vi "HAGAR-V.vi"() -> ()   [LabVIEW 2017]
uses:
  <vilib>/rvi/interface/nirviReadWriteControl/nirviReadWriteControl.xnode
  gvbooleschRT.vi
  <vilib>/rvi/interface/nirviCloseFPGA/nirviCloseFPGA.xnode
  GVMWHorst.vi
  GVMethodenwechsel.vi
  GVHorstSP.vi
  GVZwangs.vi
  GVHK1Hz.vi
  GVHeizenLH.vi
  GVAIs.vi
  GVTrapsMachs.vi
  GVaktuelleTDMS.vi
  GVECDs.vi
  GVZeitenZyklen.vi
  GVProbenvol.vi
  GVVentilposition.vi
  <vilib>/rvi/interface/nirviMethod/nirviMethod.xnode
  GVChroms.vi
  GVMetavariablen.vi
  GVZwangsMPV.vi
  Licor-Steuerung/HAGAR V/Licor-Steuerung/control/Emulate Licor output GV.vi
  Licor-Steuerung/HAGAR V/Licor-Steuerung/Licor-Steuerung.lvlib
  FPGA/FPGA-Programm-05-17.vi
  <vilib>/NI_Real-Time Target Support.lvlib
  <vilib>/FPGAPlugInAG/cRIO-9114/niLvFpga_WriteFifo_cRIO-9114.vi
  <vilib>/rvi/errors/niLvFpgaMergeErrorWithErrorCode.vi
  FPGA Bitfiles/HAGAR-V_FPGATarget_FPGA-Programm-05_gdVwCsZS6sg.lvbitx
  NiFpgaLv.dll
  <vilib>/Utility/error.llb/Error Cluster From Error Code.vi
  <vilib>/rvi/errors/niLvFpgaAdjustHostInterfaceError.vi
  <vilib>/FPGAPlugInAG/cRIO-9114/niLvFpga_Close_cRIO-9114.vi
  Licor-Steuerung/HAGAR V/Licor-Steuerung/control/Licor-Sequences.ctl
  Licor-Steuerung/HAGAR V/Licor-Steuerung/display/GUI_Cluster_Graph.ctl
  Licor-Steuerung/HAGAR V/Licor-Steuerung/control/Licor-Commands.ctl
  Licor-Steuerung/HAGAR V/Licor-Steuerung/control/Licor-Pump.ctl
  Licor-Steuerung/LicorLI7000/conventions/Licor-Source.ctl
  Licor-Steuerung/LicorLI7000/LicorLI7000.lvlib
  Licor-Steuerung/HAGAR V/Licor-Steuerung/control/Licor-Parameter.ctl
  Licor-Steuerung/HAGAR V/Licor-Steuerung/display/GUI_Cluster_Parameter.ctl
  Licor-Steuerung/HAGAR V/Licor-Steuerung/display/GUI_Cluster_sdv.ctl
panel:
  in  "Zyklus":enum16{"Mod0", "Mod1", "Mod2A", "Mod2B"}(ring)=enum."Mod1"
  in  "am Ende benutzen":bool
  in  "Methode speichern":bool
  out "ZyklusNummernGesamt":i32[](array[numeric])
  in  "veränderte Methode benutzen":bool
  in  "Methode verändern":bool
  out "ZyklusNummern":i32[](array[numeric])
  out "Big Ben, Methodenzeit, Zykluszeit0, Zykluszeit1, Zykluszeit2A, Zykluszeit2B":i32[](array[numeric])
  in  "global stop RT":bool
  in  "Methode":i32(ring) items=["Bedingsmethode", "Startmethode", "Meßmodus", "Shut-up-Methode", "Test", "HAG2 1/2", "Startmethode", "HAG2 1/2 Aufwärmen", "LicorDruckProfil1", "LicorDruckProfil2", "LicorDruckProfil0", "LicorDruckProfil3", "Kalibration-Meßmodus", "Kalibration-Meßmodus-II"]
  in  "Registerkarte":T1(tab)
  out "SHOK?":bool[](array[boolean])
  out "schnelle Heizungen":string[](array[string])
  out "schnelle Heizungen":dbl[](array[numeric])
  out "HorstOK?":bool[](array[boolean])
  out "AIs3OK?":bool[](array[boolean])
  out "AIs1OK?":bool[](array[boolean])
  out "AIs1":dbl[](array[numeric])
  out "AIs1":string[](array[string])
  out "AIs2":string[](array[string])
  out "AIs3":string[](array[string])
  out "AIs2":dbl[](array[numeric])
  out "AIs3":dbl[](array[numeric])
  out "Metavariablen":string[](array[string])
  out "MVWerte":dbl[](array[numeric])
  out "MWHorst":dbl[](array[numeric])
  out "HorstRegler":string[](array[string])
  out "AIs2OK?":bool[](array[boolean])
  out "Ventilposition":i32=1 min=1 max=6 step=1
  out "MVOK?":bool[](array[boolean])
  out "CPU Total (%)":dbl
  in  "MVFixwert":dbl[](array[numeric])
  in  "MVFix?":bool[](array[boolean])
  in  "LH-Gruppe":bool[](array[boolean])=[FALSE, FALSE, FALSE, FALSE, FALSE, FALSE, FALSE, FALSE, FALSE, FALSE, FALSE, FALSE]
  out "LangsameHeizungen":string[](array[string])
  out "Housekeeping1":cluster{dbl[], dbl[]}(graph)
  in  "Zeitachse1":i32(ring)=1 items=["Zykluszeit [s] Mod0", "Zykluszeit [s] Mod1", "Zykluszeit [s] Mod2A", "Zykluszeit [s] Mod2B"]
  in  "dargestellte Größe 1":i32(ring)=1 items=["T1-Spare1", "T1-Spare2", "T1-StirlingKühlkopf [°C]", "T1-PreCol1 [°C]", "T1-PreCol2 [°C]", "T1-MainCol1a [°C]", "T1-MainCol1b [°C]", "T1-MainCol2a [°C]", "T1-MainCol2b [°C]", "T1-BronkhorstUntena [°C]", "T1-BronkhorstUntenb [°C]", "T1-BronkhorstObena [°C]", "T1-BronkhorstObenb [°C]", "T1-2Pos1B [°C]", "T1-Spare9", "T1-2Pos1A [°C]", "T1-Spare10", "T1-TurboPump [°C]", "T1-StirlingPlatine [°C]", "T1-Spare5", "T1-Spare6", "T1-Spare7", "T1-Inlet [°C]", "F1-MFM-Spare", "F1-MFM0D [mL]", "P1-HeliumHP [bara]", "P1-HeliumLP [bara]", "P1-PumpVordruck [mbara]", "TurboSpeed", "I1-MS-AC [A]", "I1-Trap1 [A]", "I1-Trap2 [A]", "T2-ECD1a", "T2-ECD1b", "T2-ECD2a", "T2-ECD2b", "T2-Col1a", "T2-Col1b", "T2-Col2a", "T2-Col2b", "T2-Spare1", "T2-Spare2", "T2-Spare3", "T2-Spare4", "T2-Spare5", "T2-Spare6", "T2-Spare7", "F2-MFM2A", "F2-MFM2B", "F2-MFM2C", "P2-N2O_HP", "P2-N2O_LP", "P2-CO2_HP", "P2-CO2_LP", "AI-Spare1", "FL-MFM1000mL", "AI-Spare3", "AI-Spare4", "StirlingAlarm", "StirlingEmerg.", "AI-Spare7", "AI-Spare8", "AI-Spare9", "FL-MFM30mL", "T0-DC/DC5", "I0-24V_M0", "I0-48V_M1", "I0-24V_M1", "I0-28V_M2", "T0-Spare3", "T0-Spare2", "T0-Spare4", "T0-DC/DC7", "I0-20V_Laptop", "I0-28V_M1", "I0-24V_M2", "I0-12V_Licor", "T0-Spare1", "T0-Drier", "T0-Spare5", "F0-MFM0A [L]", "TL-Licor_a", "P0-Span-HP", "P0-spare1", "P0-Stickstoff-LP", "P0-Helium-LP", "P0-Cal-HP", "P0-P9Tavco[bar]", "F0-MFM0B [L]", "TL-Licor_b", "P0-Span-LP", "P0-spare2", "P0-Stickstoff-HP", "P0-Helium-HP", "P0-Cal-LP", "F0-MFM3", "Trap1 [°C]", "Trap2 [°C]", "PreCol1 [°C]", "PreCol2 [°C]", "MainCol1 [°C]", "MainCol2 [°C]", "PrC0 [bara]", "PrC0-Licor [bara]", "PrC1-Säule1 [bara]", "PrC1-Säule2 [bara]", "MFC1-Sample [ml/min]", "PrC1-BackFlush1 [bara]", "PrC1-BackFlush2 [bara]", "MFC1-Reaktant [l/min]", "MFC2A[ml/min]", "MFC2B[ml/min]", "MFC2C[ul/min]", "PrC2A[bara]", "MFC2D[ml/min]", "MFC2E[ml/min]", "PrC2B[bara]"]
  out "Housekeeping2":cluster{dbl[], dbl[]}(graph)
  in  "Zeitachse2":i32(ring)=1 items=["Zykluszeit [s] Mod0", "Zykluszeit [s] Mod1", "Zykluszeit [s] Mod2A", "Zykluszeit [s] Mod2B"]
  in  "dargestellte Größe 2":i32(ring)=1 items=["T1-Spare1", "T1-Spare2", "T1-StirlingKühlkopf [°C]", "T1-PreCol1 [°C]", "T1-PreCol2 [°C]", "T1-MainCol1a [°C]", "T1-MainCol1b [°C]", "T1-MainCol2a [°C]", "T1-MainCol2b [°C]", "T1-BronkhorstUntena [°C]", "T1-BronkhorstUntenb [°C]", "T1-BronkhorstObena [°C]", "T1-BronkhorstObenb [°C]", "T1-2Pos1B [°C]", "T1-Spare9", "T1-2Pos1A [°C]", "T1-Spare10", "T1-TurboPump [°C]", "T1-StirlingPlatine [°C]", "T1-Spare5", "T1-Spare6", "T1-Spare7", "T1-Inlet [°C]", "F1-MFM-Spare", "F1-MFM0D [mL]", "P1-HeliumHP [bara]", "P1-HeliumLP [bara]", "P1-PumpVordruck [mbara]", "TurboSpeed", "I1-MS-AC [A]", "I1-Trap1 [A]", "I1-Trap2 [A]", "T2-ECD1a", "T2-ECD1b", "T2-ECD2a", "T2-ECD2b", "T2-Col1a", "T2-Col1b", "T2-Col2a", "T2-Col2b", "T2-Spare1", "T2-Spare2", "T2-Spare3", "T2-Spare4", "T2-Spare5", "T2-Spare6", "T2-Spare7", "F2-MFM2A", "F2-MFM2B", "F2-MFM2C", "P2-N2O_HP", "P2-N2O_LP", "P2-CO2_HP", "P2-CO2_LP", "AI-Spare1", "FL-MFM1000mL", "AI-Spare3", "AI-Spare4", "StirlingAlarm", "StirlingEmerg.", "AI-Spare7", "AI-Spare8", "AI-Spare9", "FL-MFM30mL", "T0-DC/DC5", "I0-24V_M0", "I0-48V_M1", "I0-24V_M1", "I0-28V_M2", "T0-Spare3", "T0-Spare2", "T0-Spare4", "T0-DC/DC7", "I0-20V_Laptop", "I0-28V_M1", "I0-24V_M2", "I0-12V_Licor", "T0-Spare1", "T0-Drier", "T0-Spare5", "F0-MFM0A [L]", "TL-Licor_a", "P0-Span-HP", "P0-spare1", "P0-Stickstoff-LP", "P0-Helium-LP", "P0-Cal-HP", "P0-P9Tavco[bar]", "F0-MFM0B [L]", "TL-Licor_b", "P0-Span-LP", "P0-spare2", "P0-Stickstoff-HP", "P0-Helium-HP", "P0-Cal-LP", "F0-MFM3", "Trap1 [°C]", "Trap2 [°C]", "PreCol1 [°C]", "PreCol2 [°C]", "MainCol1 [°C]", "MainCol2 [°C]", "PrC0 [bara]", "PrC0-Licor [bara]", "PrC1-Säule1 [bara]", "PrC1-Säule2 [bara]", "MFC1-Sample [ml/min]", "PrC1-BackFlush1 [bara]", "PrC1-BackFlush2 [bara]", "MFC1-Reaktant [l/min]", "MFC2A[ml/min]", "MFC2B[ml/min]", "MFC2C[ul/min]", "PrC2A[bara]", "MFC2D[ml/min]", "MFC2E[ml/min]", "PrC2B[bara]"]
  out "Detektor 2":cluster{dbl[], dbl[]}[](graph)
  in  "Detektor":i32(ring) items=["ECD1", "ECD2"]
  in  "HK1YMin":dbl
  in  "HK1YMax":dbl=100.0
  in  "HK2YMin":dbl
  in  "HK2YMax":dbl=100.0
  in  "DetYMin":dbl
  in  "DetYMax":dbl=100.0
  in  "NeuerRefstrom":bool
  in  "RefStromECD1":i16=800 min=0 max=2500 step=1
  in  "RefStromECD2":i16=2100 min=0 max=2500 step=1
  out "schnelleAnzeige":cluster{dbl[], dbl[]}(graph)
  in  "TafelWischen!":bool
  in  "dargestellte Größe 3":i32(ring)=1 items=["Trap1 [°C]", "Trap2 [°C]", "PreCol1 [°C]", "PreCol2 [°C]", "MainCol1 [°C]", "MainCol2 [°C]", "PrC0 [bara]", "PrC0-Licor [bara]", "PrC1-Säule1 [bara]", "PrC1-Säule2 [bara]", "MFC1-Sample [ml/min]", "PrC1-BackFlush1 [bara]", "PrC1-BackFlush2 [bara]", "MFC1-Reaktant [l/min]", "MFC2A[ml/min]", "MFC2B[ml/min]", "MFC2C[ul/min]", "PrC2A[bara]", "MFC2D[ml/min]", "MFC2E[ml/min]", "PrC2B[bara]"]
  in  "An/Aus":bool
  in  "Registerkarte 2":T2(tab)
  in  "GUI_Cluster_Graph":T3={"time (global)"=0.0, "command queue"=[], "Rohdaten"=[], "Graph"={"X"=[], "Y"=[]}, "Manuelle Steuerung"={"Sequenz"=enum."test", "Manuelle Steuerung An/Aus"=FALSE}, "Sequenz out"={"sequence"=enum."WAIT", "Zeitpunkt next"=0.0, "delta t"=0.0}} caption="Cluster" {"Sequenz out"."Zeitpunkt next" format="%<%H:%M:%S%3u>T"; "time (global)" format="%<%H:%M:%S%3u\n%m/%d/%y>T"}
  in  "GUI_Cluster_Parameter":T5={"warmup (sequence)"=[{"time"=60, "Enum"=enum."wait"}], "calibrate S (sequence)"=[{"time"=60, "Enum"=enum."wait"}, {"time"=2, "Enum"=enum."getCalibrationParameter"}, {"time"=8, "Enum"=enum."calibration-S-CO2"}, {"time"=2, "Enum"=enum."getCalibrationParameter"}], "calibrate Z (sequence)"=[{"time"=60, "Enum"=enum."wait"}, {"time"=2, "Enum"=enum."getCalibrationParameter"}, {"time"=8, "Enum"=enum."calibration-Z-H2O"}, {"time"=2, "Enum"=enum."getCalibrationParameter"}, {"time"=8, "Enum"=enum."calibration-Z-CO2"}, {"time"=2, "Enum"=enum."getCalibrationParameter"}], "initialize (sequence)"=[{"time"=30, "Enum"=enum."wait"}, {"time"=2, "Enum"=enum."setPumpSlow"}, {"time"=2, "Enum"=enum."setPumpMedium"}, {"time"=2, "Enum"=enum."setPumpFast"}, {"time"=10, "Enum"=enum."initialize"}, {"time"=4, "Enum"=enum."getCalibrationParameter"}, {"time"=2, "Enum"=enum."resetH2O"}, {"time"=4, "Enum"=enum."resetCO2"}, {"time"=4, "Enum"=enum."getCalibrationParameter"}, {"time"=2, "Enum"=enum."setZeroParameter"}, {"time"=4, "Enum"=enum."getCalibrationParameter"}, {"time"=2, "Enum"=enum."setReference"}, {"time"=4, "Enum"=enum."getLicorTime"}, {"time"=5, "Enum"=enum."getInfo"}], "Licor-parameter"={"CO2 ref"=378.15, "CO2 span"=401.67, "H2O ref"=0.0, "H2O span"=0.0, "Zi"=1.2, "Zt"=6.494e-05, "Zm"=0.0, "S"=1.34, "Temp [C]"=45.0, "Pressure [hPa]"=1050.0, "Licor-Sources"=["CO2A W", "CO2B W", "H2OA W", "H2OB W", "T C", "T V", "P kPa", "P V", "RH %"], "Licor-Pump"="Off", "Zeitstempel"=timestamp(0 s since 1904-01-01)}} {"Licor-parameter"."Pressure [hPa]" format="%_5g"; "Licor-parameter"."Temp [C]" format="%.2f"; "Licor-parameter"."CO2 ref" format="%.2f"; "Licor-parameter"."CO2 span" format="%.2g"; "Licor-parameter"."H2O ref" format="%.2g"; "Licor-parameter"."H2O span" format="%.2g"; "Licor-parameter"."Zt" format="%#_4g"}
  in  "GUI_Cluster_sdv":T10={"Graph_sdv"={"X"=[], "Y"=[]}, "Breite"=20, "Berechnen"=FALSE, "residue"=0.0} {"residue" format="%_6g"}
  in  "VISA resource name":refnum<visa-resource-name>="ASRL1::INSTR" caption="VISA-Ressourcenname"
  out "TDMSwriteECD":errorcluster
  out "AIsFIFOread":errorcluster
  out "MWTrapsMachs":errorcluster
  out "TDMSwriteHK":errorcluster
  out "TDMScloseHK":errorcluster
  out "TDMSopenHK":errorcluster
  out "TDMScloseECD2":errorcluster
  out "TDMSopenECD2":errorcluster
  out "TDMScloseECD1":errorcluster
  out "TDMSopenECD1":errorcluster
  out "FIFOwriteRS485":errorcluster
  out "SerielleKomm.":errorcluster
  out "LH":errorcluster
  out "Zyklus":errorcluster
  out "ECD1dataBackup":errorcluster
  out "ECD2dataBackup":errorcluster
  # "Zyklen:   ===>>"
  # "MS"
  # "ECD1"
  # "ECD2"
  # "Zykluszeiten:   ===>>"
  # "MS"
  # "ECD1"
  # "ECD2"
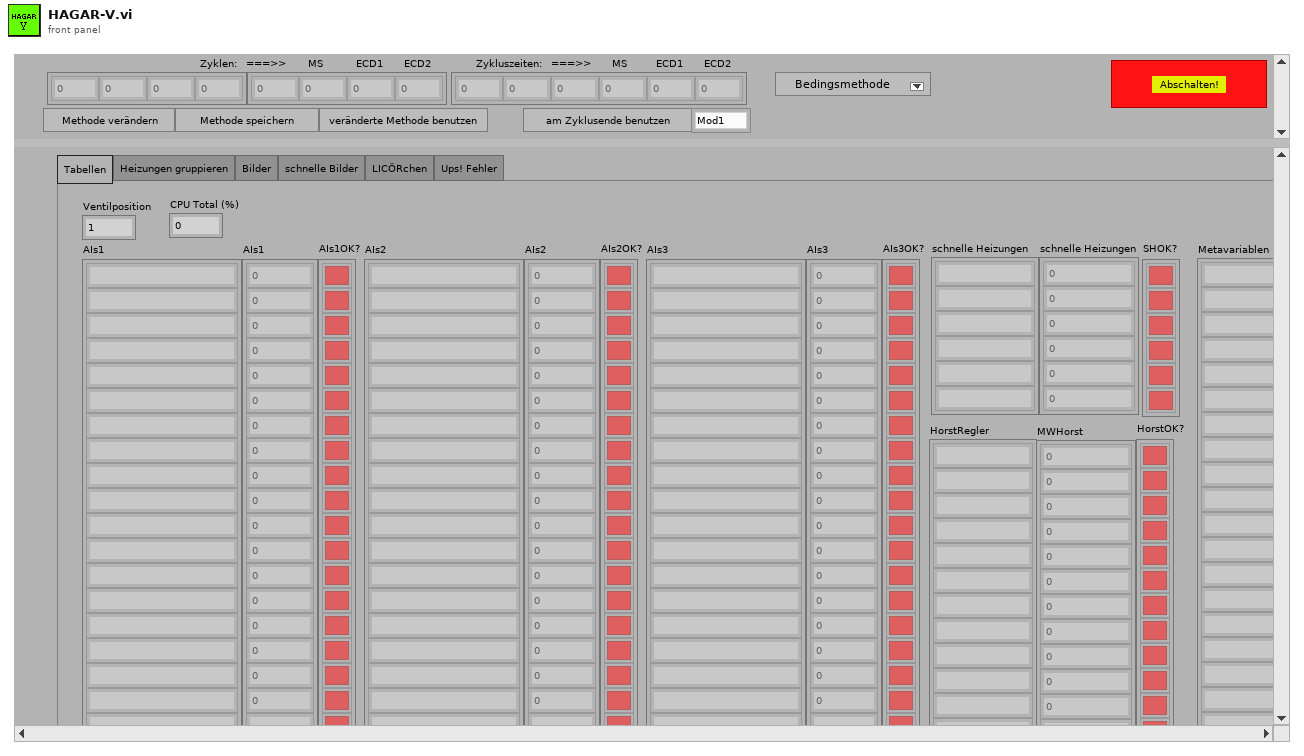
[diagram p1: front panel]
types:
  T1 = enum32{"Tabellen", "Heizungen gruppieren", "Bilder", "schnelle Bilder", "LICÖRchen", "Ups! Fehler"}
  T2 = enum32{"Graph", "Parameter / Sequenzen", "sdv", "debug"}
  T3 = typedef "Licor-Steuerung.lvlib/GUI_Cluster_Graph.ctl" = cluster{"time (global)":dbl, "command queue":cluster{"Zeit [s]":i32, "Befehl":string}[], "Rohdaten":string[], "Graph":cluster{"X":dbl[], "Y":dbl[]}, "Manuelle Steuerung":cluster{"Sequenz":T4, "Manuelle Steuerung An/Aus":bool}, "Sequenz out":cluster{"sequence":T4, "Zeitpunkt next":dbl, "delta t":dbl}}
  T4 = typedef "Licor-Steuerung.lvlib/Licor-Sequences.ctl" = enum16{"test", "WAIT", "warmup", "initialize", "calibrate Z", "calibrate S"}
  T5 = typedef "Licor-Steuerung.lvlib/GUI_Cluster_Parameter.ctl" = cluster{"warmup (sequence)":cluster{"time":i32, "Enum":T6}[], "calibrate S (sequence)":cluster{"time":i32, "Enum":T6}[], "calibrate Z (sequence)":cluster{"time":i32, "Enum":T6}[], "initialize (sequence)":cluster{"time":i32, "Enum":T6}[], "Licor-parameter":T7}
  T6 = typedef "Licor-Steuerung.lvlib/Licor-Commands.ctl" = enum16{"wait", "initialize", "resetCO2", "resetH2O", "getReference", "setReference", "calibration-Z-CO2", "calibration-Z-H2O", "calibration-S-CO2", "calibration-S-H2O", "getCalibrationParameter", "setZeroParameter", "setLicorTime", "getLicorTime", "setPumpFlowrate", "setPumpSlow", "setPumpMedium", "setPumpFast", "getInfo"}
  T7 = typedef "Licor-Steuerung.lvlib/Licor-Parameter.ctl" = cluster{"CO2 ref":dbl, "CO2 span":dbl, "H2O ref":dbl, "H2O span":dbl, "Zi":dbl, "Zt":dbl, "Zm":dbl, "S":dbl, "Temp [C]":dbl, "Pressure [hPa]":dbl, "Licor-Sources":T8[], "Licor-Pump":T9, "Zeitstempel":timestamp}
  T8 = typedef "LicorLI7000.lvlib/Licor-Source.ctl" = string
  T9 = typedef "Licor-Steuerung.lvlib/Licor-Pump.ctl" = string
  T10 = typedef "Licor-Steuerung.lvlib/GUI_Cluster_sdv.ctl" = cluster{"Graph_sdv":cluster{"X":dbl[], "Y":dbl[]}, "Breite":i32, "Berechnen":bool, "residue":dbl}
  T11 = cluster{"Zykluslängen [s]":dbl[], "ZeitpktDIOsMod0":dbl[], "ZeitpktDIOsMod1":dbl[], "ZeitpktDIOsMod2A":dbl[], "ZeitpktDIOsMod2B":dbl[], "DIOsSPMod0":bool[][], "DIOsSPMod1":bool[][], "DIOsSPMod2A":bool[][], "DIOsSPMod2B":bool[][], "Mod0HorstZeitpkt":dbl[], "Mod1HorstZeitpkt":dbl[], "Mod2AHorstZeitpkt":dbl[], "Mod2BHorstZeitpkt":dbl[], "HorstSPMod0":dbl[][], "HorstSPMod1":dbl[][], "HorstSPMod2A":dbl[][], "HorstSPMod2B":dbl[][], "LHSetpoints":dbl[], "LHHeizen?":bool[], "ZPktFPGABoolesch":dbl[], "FPGABoolesch":bool[][], "ZeitpktFPGAPID":dbl[], "FPGAPID":cluster{"d0":fxp<+/-,18,18>, "d1":fxp<+/-,21,21>}[][], "ZeitpktFPGAFixp":dbl[], dbl[][], "t_PreMach1":dbl[], "T_PreMach1":dbl[], "t_PreMach2":dbl[], "T_PreMach2":dbl[], "PIDs für \"träge\" Heizungen":cluster{"proportional gain (Kc)":dbl, "integral time (Ti, min)":dbl, "derivative time (Td, min)":dbl}[], "Zwangsbedingungen":dbl[][], "Dateien fürs MS schicken?":bool, "ZeitpunkteMPV":dbl[], "SPMPV":i32[], "ZeitpktMS-1":dbl, "ZeitpktMS-2":dbl, "Int.Start1":dbl, "Int.Stop1":dbl, "Int.Start2":dbl, "Int.Stop2":dbl, "Methodenname":string, "t_MainMach1":dbl[], "T_MainMach1":dbl[], "t_MainMach2":dbl[], "T_MainMach2":dbl[]}[]
  T12 = cluster{"DIOsMod0Nr":i32[], "DIOsMod1Nr":i32[], "DIOsMod2ANr":i32[], "DIOsMod2BNr":i32[], "AIsLH":i32[], "AnzahlRegler/Modul":i32[], "Regler für den Probenfluß":i32, "SPvorgebenMod0":string[], "SPvorgebenMod1":string[], "SPvorgebenMod2A":string[], "SPvorgebenMod2B":string[], "MWAntwortMod0":string[], "MWAntwortMod1":string[], "MWAntwortMod2A":string[], "MWAntwortMod2B":string[], "FaktorMod0":dbl[], "FaktorMod1":dbl[], "FaktorMod2A":dbl[], "FaktorMod2B":dbl[], "MWabfragenMod0":string[], "MWabfragenMod1":string[], "MWabfragenMod2A":string[], "MWabfragenMod2B":string[], "Modul1/AI koeff":dbl[][], "Modul2/AI koeff":dbl[][], "Modul3/AI koeff":dbl[][], "Traps/MachsKoeff T(R)":dbl[][], "Modul1/AIsNamen":string[], "Modul2/AIsNamen":string[], "Modul3/AIsNamen":string[], "DIOsMod0Name":string[], "DIOsMod1Name":string[], "DIOsMod2AName":string[], "DIOsMod2BName":string[], "ReglerNameMod0":string[], "ReglerNameMod1":string[], "ReglerNameMod2A":string[], "ReglerNameMod2B":string[], "Startmethode":i32, "Dateiordner Housekeeping":path, "Dateiname Housekeeping":string, "DateiordnerECD1":path, "DateinameECD1":string, "DateiordnerECD2":path, "DateinameECD2":string, "LangsameHeizungen":string[], "ModuleLH":i32[], "Metavariablen":string[], "Modul1/AI sicherer Bereich":dbl[][], "Modul2/AI sicherer Bereich":dbl[][], "Modul3/AI sicherer Bereich":dbl[][], "Traps/Machs sicherer Bereich":dbl[][], "ReglerMod0 sicherer Bereich":dbl[][], "ReglerMod1 sicherer Bereich":dbl[][], "ReglerMod2A sicherer Bereich":dbl[][], "ReglerMod2B sicherer Bereich":dbl[][], "Metavariablen grüner Bereich":dbl[][], "Traps/MachsKoeff R(U)":dbl[][], "LHGruppe":bool[]}
  T13 = enum16{"open", "replace", "create", "open or create", "replace or create", "replace or create with confirmation"}
  T14 = cluster{"Zyklus1":i32, "Zeitachse1":i32, "dargestellte Größe 1":i32, "Zyklus2":i32, "Zeitachse2":i32, "dargestellte Größe 2":i32}
  T15 = cluster{"DIOsMod0Name":string[], "DIOsMod1Name":string[], "DIOsMod2AName":string[], "DIOsMod2BName":string[], "ReglerNameMod0":string[], "ReglerNameMod1":string[], "ReglerNameMod2A":string[], "ReglerNameMod2B":string[], "LangsameHeizungen":string[]}
  T16 = cluster{"Zykluslängen [s]":dbl[], "ZeitpktDIOsMod0":dbl[], "ZeitpktDIOsMod1":dbl[], "ZeitpktDIOsMod2A":dbl[], "ZeitpktDIOsMod2B":dbl[], "DIOsSPMod0":bool[][], "DIOsSPMod1":bool[][], "DIOsSPMod2A":bool[][], "DIOsSPMod2B":bool[][], "Mod0HorstZeitpkt":dbl[], "Mod1HorstZeitpkt":dbl[], "Mod2AHorstZeitpkt":dbl[], "Mod2BHorstZeitpkt":dbl[], "HorstSPMod0":dbl[][], "HorstSPMod1":dbl[][], "HorstSPMod2A":dbl[][], "HorstSPMod2B":dbl[][], "LHSetpoints":dbl[], "LHHeizen?":bool[], "ZPktFPGABoolesch":dbl[], "FPGABoolesch":bool[][], "ZeitpktFPGAPID":dbl[], "FPGAPID":cluster{"d0":fxp<+/-,18,18>, "d1":fxp<+/-,21,21>}[][], "ZeitpktFPGAFixp":dbl[], dbl[][], "t_PreMach1":dbl[], "T_PreMach1":dbl[], "t_PreMach2":dbl[], "T_PreMach2":dbl[], "PIDs für \"träge\" Heizungen":cluster{"proportional gain (Kc)":dbl, "integral time (Ti, min)":dbl, "derivative time (Td, min)":dbl}[], "Zwangsbedingungen":dbl[][], "Dateien fürs MS schicken?":bool, "ZeitpunkteMPV":dbl[], "SPMPV":i32[], "ZeitpktMS-1":dbl, "ZeitpktMS-2":dbl, "Int.Start1":dbl, "Int.Stop1":dbl, "Int.Start2":dbl, "Int.Stop2":dbl, "Methodenname":string, "t_MainMach1":dbl[], "T_MainMach1":dbl[], "t_MainMach2":dbl[], "T_MainMach2":dbl[]}
  T17 = cluster{"Modul1/AI sicherer Bereich":dbl[][], "Modul2/AI sicherer Bereich":dbl[][], "Modul3/AI sicherer Bereich":dbl[][], "Traps/Machs sicherer Bereich":dbl[][], dbl[][], "Metavariablen grüner Bereich":dbl[][]}
  T18 = cluster{"created path":path, "created path":path}
  T19 = cluster{"created path":path, "created path":path, "created path":path, "Dateiname Housekeeping":string, "DateinameECD1":string, "DateinameECD2":string, "tdms0":refnum<k34>, "tdms1":refnum<k34>, "tdms0":refnum<k34>, "tdms1":refnum<k34>, "tdms0":refnum<k34>, "tdms1":refnum<k34>}
  T20 = cluster{"d0":fxp<+/-,18,18>, "d1":fxp<+/-,21,21>}[][]
  T21 = cluster{"proportional gain (Kc)":dbl, "integral time (Ti, min)":dbl, "derivative time (Td, min)":dbl}[]
  T22 = cluster{cluster{"ZeitpktDIOsMod2B":dbl[]}[], cluster{"DIOsSPMod2B":bool[][]}[], cluster{"Mod2BHorstZeitpkt":dbl[]}[], cluster{"HorstSPMod2B":dbl[][]}[], "LHHeizen?":bool[], "ZPktFPGABoolesch":dbl[], "FPGABoolesch":bool[][], "ZeitpktFPGAPID":dbl[], "FPGAPID":cluster{"d0":fxp<+/-,18,18>, "d1":fxp<+/-,21,21>}[][], "ZeitpktFPGAFixp":dbl[], dbl[][], "t_PreMach1":dbl[], "T_PreMach1":dbl[], "t_PreMach2":dbl[], "T_PreMach2":dbl[], "ZeitpunkteMPV":dbl[], "SPMPV":i32[], "t_MainMach1":dbl[], "T_MainMach1":dbl[], "t_MainMach2":dbl[], "T_MainMach2":dbl[]}
  T23 = cluster{"Zykluslängen [s]":dbl[], "ZeitpktDIOsMod0":dbl[], "ZeitpktDIOsMod1":dbl[], "ZeitpktDIOsMod2A":dbl[], "ZeitpktDIOsMod2B":dbl[], "DIOsSPMod0":bool[][], "DIOsSPMod1":bool[][], "DIOsSPMod2A":bool[][], "DIOsSPMod2B":bool[][], "Mod0HorstZeitpkt":dbl[], "Mod1HorstZeitpkt":dbl[], "Mod2AHorstZeitpkt":dbl[], "Mod2BHorstZeitpkt":dbl[], "HorstSPMod0":dbl[][], "HorstSPMod1":dbl[][], "HorstSPMod2A":dbl[][], "HorstSPMod2B":dbl[][], "LangsameHeizungenSP":dbl[], "LHHeizen?":bool[], "ZPktFPGABoolesch":dbl[], "FPGABoolesch":bool[][], "ZeitpktFPGAPID":dbl[], "FPGAPID":cluster{"d0":fxp<+/-,18,18>, "d1":fxp<+/-,21,21>}[][], "ZeitpktFPGAFixp":dbl[], "FPGAFixp":dbl[][], "t_PreMach1":dbl[], "T_PreMach1":dbl[], "t_PreMach2":dbl[], "T_PreMach2":dbl[], "PIDs für \"träge\" Heizungen":cluster{"proportional gain (Kc)":dbl, "integral time (Ti, min)":dbl, "derivative time (Td, min)":dbl}[], "Zwangsbedingungen":dbl[][], "MS-Daten?":bool, "ZeitpunkteMPV":dbl[], "SetpointMPV":i32[], "ZeitpktMS-1":dbl, "ZeitpktMS-2":dbl, "Int.Start1":dbl, "Int.Stop1":dbl, "Int.Start2":dbl, "Int.Stop2":dbl, "Methodenname":string, "t_MainMach1":dbl[], "T_MainMach1":dbl[], "t_MainMach2":dbl[], "T_MainMach2":dbl[]}
  T24 = cluster{"ZyklusNummern":i32[], "ZeilennummernDIOs":i32[], "ZwangsDIO?":cluster{bool[]}[], "ZeilennummernHorst":i32[], "ZwangsHorst?":cluster{bool[]}[], "ZeileFPGABoolesch":i32, "ZwangsFPGABoolesch?":bool[], "ZeileFPGAPID":i32, "ZeileFPGAFixp":i32, "ZeilePreMach1":i32, "ZeilePreMach2":i32, "ZeilennummerMPV":i32, "ZeileMainMach1":i32, "ZeileMainMach2":i32, "ZwangsMPV?":bool}
  T25 = typedef "NI_Real-Time Target Support.lvlib/RT CPU Load.ctl" = cluster{"Total (%)":dbl, "Time Critical (%)":dbl, "Timed Structures (%)":dbl, "High (%)":dbl, "Above Normal (%)":dbl, "Normal (%)":dbl, "Background (%)":dbl, "Idle (%)":dbl, "ISR (%)":dbl}
  T26 = cluster{"ZyklusNummern":i32[], i32[], "ZwangsDIO?":cluster{bool[]}[], i32[], "ZwangsHorst?":cluster{bool[]}[], i32, "ZwangsFPGABoolesch?":bool[], i32, i32, "ZeileMach":i32, "ZeileMach":i32, i32, "ZeileMach":i32, "ZeileMach":i32, "ZwangsMPV?":bool}
  T27 = cluster{string[], string[], string[], dbl[], dbl[], dbl[]}
  T28 = cluster{"Befehle1":string[], "Befehle2":string[], "Befehle3":string[]}
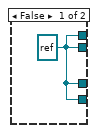
[diagram p2: hidden frame]
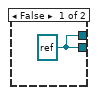
[diagram p3: hidden frame]
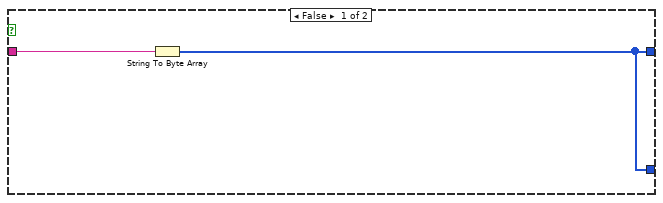
[diagram p6: hidden frame]
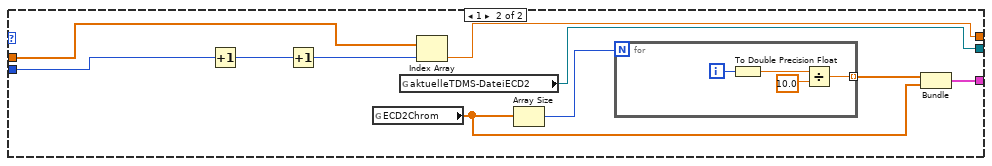
[diagram p16: hidden frame]
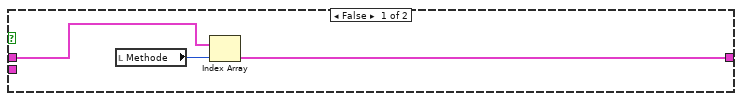
[diagram p17: hidden frame]
diagram:
  w2 = path "c:/methoden.pery" ("Datei (Dialog verwenden)")
  w3 = path "c:/einstellungen.pery" ("Datei (Dialog verwenden)")
  n1 = Open/Create/Replace File(file path (use dialog)=w3, operation (0:open)=T13."open" ("Operation (0:Öffnen)")) -> (refnum out=w15:refnum<file>)  [unwired: 4 in, 2 out]
  n2 = Open/Create/Replace File(file path (use dialog)=w2, operation (0:open)=T13."open" ("Operation (0:Öffnen)")) -> (refnum out=w11:refnum<file>)  [unwired: 4 in, 2 out]
  n3 = Read from Binary File(5:T12 {"DIOsMod0Nr"=[], "DIOsMod1Nr"=[], "DIOsMod2ANr"=[], "DIOsMod2BNr"=[], "AIsLH"=[], "AnzahlRegler/Modul"=[], "Regler für den Probenfluß"=0, "SPvorgebenMod0"=[], "SPvorgebenMod1"=[], "SPvorgebenMod2A"=[], "SPvorgebenMod2B"=[], "MWAntwortMod0"=[], "MWAntwortMod1"=[], "MWAntwortMod2A"=[], "MWAntwortMod2B"=[], "FaktorMod0"=[], "FaktorMod1"=[], "FaktorMod2A"=[], "FaktorMod2B"=[], "MWabfragenMod0"=[], "MWabfragenMod1"=[], "MWabfragenMod2A"=[], "MWabfragenMod2B"=[], "Modul1/AI koeff"=[], "Modul2/AI koeff"=[], "Modul3/AI koeff"=[], "Traps/MachsKoeff T(R)"=[], "Modul1/AIsNamen"=[], "Modul2/AIsNamen"=[], "Modul3/AIsNamen"=[], "DIOsMod0Name"=[], "DIOsMod1Name"=[], "DIOsMod2AName"=[], "DIOsMod2BName"=[], "ReglerNameMod0"=[], "ReglerNameMod1"=[], "ReglerNameMod2A"=[], "ReglerNameMod2B"=[], "Startmethode"=0, "Dateiordner Housekeeping"=path "", "Dateiname Housekeeping"="", "DateiordnerECD1"=path "", "DateinameECD1"="", "DateiordnerECD2"=path "", "DateinameECD2"="", "LangsameHeizungen"=[], "ModuleLH"=[], "Metavariablen"=[], "Modul1/AI sicherer Bereich"=[], "Modul2/AI sicherer Bereich"=[], "Modul3/AI sicherer Bereich"=[], "Traps/Machs sicherer Bereich"=[], "ReglerMod0 sicherer Bereich"=[], "ReglerMod1 sicherer Bereich"=[], "ReglerMod2A sicherer Bereich"=[], "ReglerMod2B sicherer Bereich"=[], "Metavariablen grüner Bereich"=[], "Traps/MachsKoeff R(U)"=[], "LHGruppe"=[]} ("output cluster"), 11:w15) -> (2:w13:T12, 3:w14:refnum<file>)  [unwired: 4 in, 2 out]
  n4 = Read from Binary File(5:T11 [], 11:w11) -> (2:w9:T11, 3:w10:refnum<file>)  [unwired: 4 in, 2 out]
  n5 = Close File(refnum=w14) -> ()  [unwired: 1 in, 2 out]
  n6 = Close File(refnum=w10) -> ()  [unwired: 1 in, 2 out]
  n7 = flat-sequence {
    tunnel: [w84] -> w42
    tunnel: [w145] -> w41
    tunnel: [w88] -> w39
    tunnel: [w278] -> w38
    tunnel: [w280] -> w37
    tunnel: [w272] -> w36
    tunnel: [w279] -> w35
    tunnel: [w202] -> w34
    tunnel: [w271] -> w33
    tunnel: [w270] -> w32
    tunnel: [w264] -> w31
    tunnel: [w205] -> w30
    tunnel: [w179] -> w29
    tunnel: [w277] -> w28
    tunnel: [w269] -> w27
    tunnel: [w268] -> w26
    tunnel: [w260] -> w25
    tunnel: [w259] -> w24
    tunnel: [w258] -> w23
    tunnel: [w257] -> w22
    tunnel: [w256] -> w21
    tunnel: [w255] -> w20
    tunnel: [w252] -> w19
    tunnel: [w234] -> w18
    tunnel: w13 -> [w127]
    tunnel: [w233] -> w17
    tunnel: w9 -> [w146]
    tunnel: [w145] -> w8
    tunnel: [w127] -> w7
    tunnel: [w96] -> w6
    tunnel: w3 -> [w81]
    tunnel: w2 -> [w77]
    tunnel: [w58] -> w1
    tunnel: w42 -> [w346]
    tunnel: w41 -> [w419]
    tunnel: [w346] -> w40
    tunnel: w39 -> [_]
    tunnel: w38 -> [w377]
    tunnel: w37 -> [w376]
    tunnel: w36 -> [w378]
    tunnel: w35 -> [w375]
    tunnel: w34 -> [w350]
    tunnel: w33 -> [w345]
    tunnel: w32 -> [w342]
    tunnel: w31 -> [w339]
    tunnel: w30 -> [w340]
    tunnel: w29 -> [w343]
    tunnel: w28 -> [w417]
    tunnel: w27 -> [w348]
    tunnel: w26 -> [w418]
    tunnel: w25 -> [w321]
    tunnel: w24 -> [w320]
    tunnel: w23 -> [w319]
    tunnel: w22 -> [w415]
    tunnel: w21 -> [w414]
    tunnel: w20 -> [w413]
    tunnel: w19 -> [w367]
    tunnel: w18 -> [w349]
    tunnel: w17 -> [w338]
    tunnel: w9 -> [w337]
    tunnel: w8 -> [w335]
    tunnel: w7 -> [_]
    tunnel: w6 -> [w314]
    tunnel: w1 -> [w313]
    tunnel: w40 -> [w1215]
    frame #0 {
      w54 = "config" ("string")
      w76 = string[] ["Trap1 [°C]", "Trap2 [°C]", "PreCol1 [°C]", "PreCol2 [°C]", "MainCol1 [°C]", "MainCol2 [°C]"]
      w147 = TRUE
      w161 = 0.0 ("Probenvol.1")
      w168 = dbl[] [-1.0] ("ECD1MW")
      w169 = FALSE ("ECD1Empfangen?")
      w275 = string[] ["Big Ben [s]", "Methodenzeit [s]", "Zykluszeit [s] Mod0", "Zykluszeit [s] Mod1", "Zykluszeit [s] Mod2A", "Zykluszeit [s] Mod2B"]
      w265 = FALSE ("Undefinierte Werte möglich")
      w266 = FALSE ("global stop RT")
      n8 = for {
        tunnel: [w308] -> w273 mode=indexing
        tunnel: w146 -> [w309] mode=indexing
        n9 = Unbundle(w309) -> ("Methodenname"=w308:string)  [unwired: 44 out]
      }
      n10 = Unbundle(w127) -> ("DIOsMod0Nr"=w189:i32[], "DIOsMod1Nr"=w188:i32[], "DIOsMod2ANr"=w187:i32[], "DIOsMod2BNr"=w186:i32[], "AIsLH"=w176:i32[], "AnzahlRegler/Modul"=w179:i32[], "Regler für den Probenfluß"=w233:i32, "SPvorgebenMod0"=w232:string[], "SPvorgebenMod1"=w231:string[], "SPvorgebenMod2A"=w230:string[], "SPvorgebenMod2B"=w229:string[], "MWAntwortMod0"=w228:string[], "MWAntwortMod1"=w227:string[], "MWAntwortMod2A"=w226:string[], "MWAntwortMod2B"=w225:string[], "FaktorMod0"=w224:dbl[], "FaktorMod1"=w223:dbl[], "FaktorMod2A"=w222:dbl[], "FaktorMod2B"=w221:dbl[], "MWabfragenMod0"=w220:string[], "MWabfragenMod1"=w219:string[], "MWabfragenMod2A"=w218:string[], "MWabfragenMod2B"=w217:string[], "Modul1/AI koeff"=w216:dbl[][], "Modul2/AI koeff"=w215:dbl[][], "Modul3/AI koeff"=w214:dbl[][], "Traps/MachsKoeff T(R)"=w213:dbl[][], "Modul1/AIsNamen"=w212:string[], "Modul2/AIsNamen"=w211:string[], "Modul3/AIsNamen"=w210:string[], "DIOsMod0Name"=w125:string[], "DIOsMod1Name"=w126:string[], "DIOsMod2AName"=w124:string[], "DIOsMod2BName"=w123:string[], "ReglerNameMod0"=w138:string[], "ReglerNameMod1"=w137:string[], "ReglerNameMod2A"=w136:string[], "ReglerNameMod2B"=w135:string[], "Startmethode"=w145:i32, "Dateiordner Housekeeping"=w63:path, "Dateiname Housekeeping"=w209:string, "DateiordnerECD1"=w68:path, "DateinameECD1"=w208:string, "DateiordnerECD2"=w60:path, "DateinameECD2"=w207:string, "LangsameHeizungen"=w206:string[], "ModuleLH"=w201:i32[], "Metavariablen"=w140:string[], "Modul1/AI sicherer Bereich"=w100:dbl[][], "Modul2/AI sicherer Bereich"=w99:dbl[][], "Modul3/AI sicherer Bereich"=w98:dbl[][], "Traps/Machs sicherer Bereich"=w97:dbl[][], "ReglerMod0 sicherer Bereich"=w95:dbl[][], "ReglerMod1 sicherer Bereich"=w94:dbl[][], "ReglerMod2A sicherer Bereich"=w93:dbl[][], "ReglerMod2B sicherer Bereich"=w92:dbl[][], "Metavariablen grüner Bereich"=w90:dbl[][], "LHGruppe"=w83:bool[])  [unwired: 1 out]
      "Metavariablen" <- w140
      "LangsameHeizungen" <- w206
      n11 = Initialize Array(0, 4 ("Dimension")) -> (w162:i32[])
      n12 = Initialize Array(0.0 ("Element"), 6 ("Dimension")) -> (w165:dbl[])
      n13 = global write "GVMethodenwechsel.vi" "Methodenwechsel?"(FALSE ("Methodenwechsel?")) -> ()
      n14 = local write "NeuerRefstrom"(FALSE ("NeuerRefstrom")) -> ()
      n15 = property on="dargestellte Größe 2" class="Ring (strikt)"("AllowUndefVals"=w265) -> ()  [unwired: 2 in, 2 out]
      n16 = property on="Zeitachse2" class="Ring (strikt)"("AllowUndefVals"=w265) -> ()  [unwired: 2 in, 2 out]
      n17 = property on="Zeitachse1" class="Ring (strikt)"("AllowUndefVals"=w265) -> ()  [unwired: 2 in, 2 out]
      n18 = property on="dargestellte Größe 1" class="Ring (strikt)"("AllowUndefVals"=w265) -> ()  [unwired: 2 in, 2 out]
      n19 = property on="Methode" class="Ring (strikt)"("AllowUndefVals"=w265) -> ()  [unwired: 2 in, 2 out]
      n20 = global write "GVProbenvol.vi" "Probenvol.1"(w161) -> ()
      n21 = global write "GVProbenvol.vi" "Probenvol.2"(w161) -> ()
      n22 = global write "GVECDs.vi" "ECD1MW"(w168) -> ()
      n23 = global write "GVECDs.vi" "ECD2MW"(w168) -> ()
      n24 = global write "GVECDs.vi" "ECD1Empfangen?"(w169) -> ()
      n25 = global write "GVECDs.vi" "ECD2Empfangen?"(w169) -> ()
      n26 = local write "global stop RT"(w266) -> ()
      n27 = global write "gvbooleschRT.vi" "global stop RT"(w266) -> ()
      n28 = global write "GVZeitenZyklen.vi" "ZyklusNummern"(w162) -> ()
      n29 = global write "GVZeitenZyklen.vi" "ZyklusNummernGesamt"(w162) -> ()
      n30 = global write "GVZeitenZyklen.vi" "Big Ben, Methodenzeit, Zykluszeit0, Zykluszeit1, Zykluszeit2A, Zykluszeit2B"(w165) -> ()
      n31 = property on="Methode" class="Ring (strikt)"("Value"=w145) -> ()  [unwired: 2 in, 2 out]
      n32 = Initialize Array(-1.0 ("Element"), 6 ("Dimension")) -> (w172:dbl[])
      n33 = Initialize Array(FALSE, 10 ("Dimension")) -> (w180:bool[])
      n34 = Initialize Array(-1.0 ("Element"), 96 ("Dimension")) -> (w173:dbl[])
      n35 = local write "LH-Gruppe"(w83) -> ()
      n36 = Strip Path(path=w63) -> (stripped path=w64:path)  [unwired: 1 out]
      n37 = Strip Path(path=w68) -> (stripped path=w65:path, name=w67:string)
      n38 = global write "GVZwangs.vi" "ZwangsFPGABoolesch!"(w180) -> ()
      n39 = global write "GVZwangs.vi" "ZwangsFPGABoolesch?"(w180) -> ()
      n40 = global write "GVTrapsMachs.vi" "Traps/Machs"(w172) -> ()
      n41 = global write "GVAIs.vi" "AIs"(w173) -> ()
      n42 = for {
        tunnel: w179 -> [w286] mode=indexing
        tunnel: [w283] -> w178 mode=indexing
        tunnel: [w281] -> w177 mode=indexing
        n43 = Initialize Array(0.0 ("Element"), w286) -> (w284:dbl[])
        n44 = Initialize Array(FALSE, w286) -> (w282:bool[])
        n45 = Bundle(w284) -> (w283:cluster{dbl[]})  [unwired: 1 in]
        n46 = Bundle(w282) -> (w281:cluster{bool[]})  [unwired: 1 in]
      }
      n47 = Bundle("DIOsMod0Name"=w125, "DIOsMod1Name"=w126, "DIOsMod2AName"=w124, "DIOsMod2BName"=w123, "ReglerNameMod0"=w138, "ReglerNameMod1"=w137, "ReglerNameMod2A"=w136, "ReglerNameMod2B"=w135, "LangsameHeizungen"=w206) -> (w268:T15)  [unwired: 1 in]
      n48 = Build Array (concatenate)(w138, w137, w136, w135) -> (w160:string[])
      n49 = Build Array (concatenate)(w228, w227, w226, w225) -> (w279:string[])
      n50 = Build Array (concatenate)(w232, w231, w230, w229) -> (w280:string[])
      n51 = Build Array (concatenate)(w224, w223, w222, w221) -> (w272:dbl[])
      n52 = Build Array (concatenate)(w220, w219, w218, w217) -> (w278:string[])
      n53 = Build Array (concatenate)(w138, w137, w136, w135) -> (→"HorstRegler":string[])
      n54 = Build Array (concatenate)(w95, w94, w93, w92) -> (w91:dbl[][])
      n55 = Array Size(array=w140) -> (size(s)=w75:i32)
      n56 = Build Array(w189, w188, w187, w186) -> (w185:i32[][])
      n57 = Array Size(array=w206) -> (size(s)=w205:i32)
      n58 = Add Array Elements(numeric array=w179) -> (sum=w264:i32)
      n59 = Array Size(array=w176) -> (size(s)=w175:i32)
      n60 = Index Array(array=w146, index=w145) -> (element=w144:T16)
      n61 = Add Array Elements(numeric array=w179) -> (sum=w191:i32)
      n62 = Decrement(x=w201) -> (x-1=w200:i32[])
      n63 = Build Cluster Array(w189, w188, w187, w186) -> (w271:cluster{"DIOsMod2BNr":i32[]}[])
      n64 = Build Array (concatenate)(w212, w211, w210) -> (w151:string[])
      n65 = Index Array(array=w213, index (col)=2 ("Deaktivierter Index (Spalte)")) -> (element=w260:dbl[])  [unwired: 1 in]
      n66 = Index Array(array=w213, index (col)=0 ("Deaktivierter Index (Spalte)")) -> (element=w258:dbl[])  [unwired: 1 in]
      n67 = Index Array(array=w213, index (col)=1 ("Deaktivierter Index (Spalte)")) -> (element=w259:dbl[])  [unwired: 1 in]
      n68 = Concatenate Strings("?SE0,SETP,0800" ("string"), "\n") -> (w102:string)
      n69 = Concatenate Strings("?SE0,SETP,2100" ("string"), "\n") -> (w109:string)
      n70 = Strip Path(path=w60) -> (stripped path=w59:path, name=w62:string)
      n71 = Concatenate Strings(w67, "Backup" ("string")) -> (w49:string)
      n72 = Build Path(base path=w64, name or relative path=w54) -> (appended path=w55:path)
      n73 = Build Path(base path=w65, name or relative path=w49) -> (appended path=w50:path)
      n74 = Concatenate Strings(w62, "Backup" ("string")) -> (w45:string)
      n75 = for {
        tunnel: w271 -> [w311] mode=indexing
        tunnel: [w312] -> w270 mode=indexing
        n76 = Unbundle(w311) -> ("DIOsMod2BNr"=w310:i32[])
        n77 = Array Size(array=w310) -> (size(s)=w312:i32)
      }
      n78 = property on="Methode" class="Ring (strikt)"("Strings []"=w273) -> ()  [unwired: 2 in, 2 out]
      n79 = Bundle("Modul1/AI sicherer Bereich"=w100, "Modul2/AI sicherer Bereich"=w99, "Modul3/AI sicherer Bereich"=w98, "Traps/Machs sicherer Bereich"=w97, w91, "Metavariablen grüner Bereich"=w90) -> (w96:T17)  [unwired: 1 in]
      n80 = Build Array (concatenate)(w173, w172) -> (w171:dbl[])
      n81 = Initialize Array(FALSE, w75) -> (w72:bool[])
      n82 = Array Size(array=w185) -> (size(s)=w184:i32[])
      n83 = Unbundle(w144) -> ("SPMPV"=w143:i32[])  [unwired: 44 out]
      n84 = Open/Create/Replace File(file path (use dialog)=path "c:/fromcriordy.txt" ("Dateipfad (Dialog verwenden)"), operation (0:open)=T13."replace or create" ("Operation (0:Öffnen)")) -> (refnum out=w237:refnum<file>, error out=w238:errorcluster)  [unwired: 4 in, 1 out]
      n85 = Initialize Array(0.0 ("element"), w75) -> (w73:dbl[])
      n86 = Initialize Array(0.0 ("Element"), w191) -> (w190:dbl[])
      n87 = Build Path(base path=w59, name or relative path=w45) -> (appended path=w44:path)
      n88 = Get Date/Time In Seconds() -> (seconds since 1Jan1904=w133:timestamp)
      n89 = Initialize Array(FALSE, w175) -> (w170:bool[])
      n90 = Multiply(x=w200, y=32) -> (x*y=w203:i32[])
      n91 = Initialize Array(-1.0, w191) -> (w193:dbl[])
      n92 = Array Subset(array=w151, index=32 ("Index"), length=32 ("Länge")) -> (→"AIs2":string[])
      n93 = Array Subset(array=w151, index=0 ("Index"), length=32 ("Länge")) -> (→"AIs1":string[])
      n94 = Array Subset(array=w151, index=64 ("Index"), length=32 ("Länge")) -> (→"AIs3":string[])
      n95 = global write "GVHK1Hz.vi" "Mod1Mod2Mod3/AITrapsMachs1Hz"(w171) -> ()
      n96 = global write "GVMetavariablen.vi" "Metavariablen"(w73) -> ()
      n97 = global write "GVHeizenLH.vi" "Heizen?LH"(w170) -> ()
      n98 = global write "GVZwangs.vi" "ZwangsLangsameHeizungenAn!"(w170) -> ()
      n99 = for {
        tunnel: w184 -> [w291] mode=indexing
        tunnel: [w288] -> w183 mode=indexing
        n100 = Initialize Array(FALSE, w291) -> (w289:bool[])
        n101 = Bundle(w289) -> (w288:cluster{bool[]})  [unwired: 1 in]
      }
      n102 = global write "GVHorstSP.vi" "HorstSP"(w190) -> ()
      n103 = global write "GVZwangs.vi" "ZwangsLangsameHeizungenAn?"(w170) -> ()
      n104 = global write "GVMetavariablen.vi" "MVFixwert"(w73) -> ()
      n105 = Add(x=w203, y=w176) -> (x+y=w202:i32[])
      n106 = Close File(refnum=w237, error in=w238) -> (path=w269:path)  [unwired: 1 out]
      n107 = Format Date/Time String(time format string (%c)="%Y-%m-%d--%H-%M" ("Zeitformatierungs-String (%c)"), seconds (now)=w133) -> (date/time string=w46:string)  [unwired: 1 in]
      n108 = Concatenate Strings(w49, w46) -> (w51:string)
      n109 = Concatenate Strings(w45, w46) -> (w47:string)
      n110 = Build Path(base path=w50, name or relative path=w51) -> (appended path=w48:path)
      n111 = Build Path(base path=w44, name or relative path=w47) -> (appended path=w43:path)
      n112 = Concatenate Strings(w54, w46) -> (w53:string)
      n113 = Create Folder(path (use dialog)=w48) -> (created path=w57:path)  [unwired: 2 in, 2 out]
      n114 = Create Folder(path (use dialog)=w43) -> (created path=w56:path)  [unwired: 2 in, 2 out]
      n115 = Bundle("created path"=w57, "created path"=w56) -> (w58:T18)  [unwired: 1 in]
      n116 = String To Byte Array(string=w102) -> (unsigned byte array=w104:u8[])
      n117 = String To Byte Array(string=w109) -> (unsigned byte array=w114:u8[])
      n118 = global write "GVMetavariablen.vi" "MVFix?"(w72) -> ()
      n119 = Index Array(array=w143, index=0) -> (element=w141:i32)
      n120 = Build Path(base path=w55, name or relative path=w53) -> (appended path=w52:path)
      n121 = call "FPGA-Start-15-07-17.vi"() -> ("error out"=w88:errorcluster, "FPGA VI Reference Out"=w87:refnum<k20>)  [unwired: 2 in]
      n122 = local write "MVFix?"(w72) -> ()
      n123 = local write "MVFixwert"(w73) -> ()
      n124 = global write "GVMWHorst.vi" "MWHorst"(w193) -> ()
      n125 = global write "GVVentilposition.vi" "Ventilposition"(w141) -> ()
      n126 = Build Array (concatenate)(string[] ["Jahr", "Monat", "Tag", "Stunde", "Minute", "Sekunde"] ("Array"), string[] ["Datei Nr.", "Methode Nr.", "Zyklusnr. Mod0", "Zyklusnr. Mod1", "Zyklusnr. Mod2A", "Zyklusnr. Mod2B"], w275, w151, w76, w160, "Probenvolumen1", "Probenvolumen2", "Ventilposition" ("element"), string[] ["CPU Total", "CPU Time critical", "CPU Timed Structures", "CPU High", "CPU Above normal", "CPU Normal", "CPU Background", "CPU Idle", "CPU ISR", "Memory", "SekundenTotalBrutal"]) -> (w277:string[])
      n127 = Build Array (concatenate)(w76, w160) -> (w159:string[])
      n128 = Build Array (concatenate)(w151, w76, w160) -> (w158:string[])
      n129 = Join Numbers(hi=w104, lo=u8 5) -> ((hi.lo)=w101:u16[])
      n130 = Join Numbers(hi=w114, lo=u8 6) -> ((hi.lo)=w112:u16[])
      n131 = Split 1D Array(array=w275, index=2 ("Index")) -> (second subarray=w267:string[])  [unwired: 1 out]
      n132 = Concatenate Strings("HK " ("String"), w46) -> (w120:string)
      n133 = Concatenate Strings("ECD1 " ("String"), w46) -> (w118:string)
      n134 = Concatenate Strings("ECD2 " ("String"), w46) -> (w116:string)
      n135 = property on="dargestellte Größe 1" class="Ring (strikt)"("Strings []"=w158) -> ()  [unwired: 2 in, 2 out]
      n136 = global write "GVZwangs.vi" "ZwangsHorst!"(w178) -> ()
      n137 = global write "GVZwangs.vi" "ZwangsHorst?"(w177) -> ()
      n138 = xnode "Invoke Method"("FPGA-VI-Referenz (Eingang)"=w87, "Daten"=w101) -> ("FPGA-VI-Referenz (Ausgang)"=w107:refnum<k20>)  [unwired: 2 in, 2 out]
      n139 = property on="dargestellte Größe 2" class="Ring (strikt)"("Strings []"=w158) -> ()  [unwired: 2 in, 2 out]
      n140 = property on="dargestellte Größe 3" class="Ring (strikt)"("Strings []"=w159) -> ()  [unwired: 2 in, 2 out]
      n141 = property on="Zeitachse2" class="Ring (strikt)"("Strings []"=w267) -> ()  [unwired: 2 in, 2 out]
      n142 = property on="Zeitachse1" class="Ring (strikt)"("Strings []"=w267) -> ()  [unwired: 2 in, 2 out]
      n143 = xnode "Invoke Method"("FPGA-VI-Referenz (Eingang)"=w107, "Daten"=w112) -> ("FPGA-VI-Referenz (Ausgang)"=w86:refnum<k20>)  [unwired: 2 in, 2 out]
      n144 = Create Folder(path (use dialog)=w52) -> (created path=w69:path)  [unwired: 2 in, 2 out]
      n145 = Build Path(base path=w63, name or relative path=w120) -> (appended path=w78:path)
      n146 = Build Path(base path=w68, name or relative path=w118) -> (appended path=w130:path)
      n147 = Build Path(base path=w60, name or relative path=w116) -> (appended path=w132:path)
      n148 = Strip Path(path=w81) -> (name=w80:string)  [unwired: 1 out]
      n149 = global write "GVZwangs.vi" "ZwangsDIO!"(w183) -> ()
      n150 = global write "GVZwangs.vi" "ZwangsDIO?"(w183) -> ()
      n151 = call "MPVSenden-15-07-17.vi"("Ventilposition"=0, "FPGA VI Reference In"=w86) -> ("FPGA VI Reference Out"=w84:refnum<k20>)  [unwired: 1 in, 2 out]
      n152 = Build Path(base path=w69, name or relative path=w80) -> (appended path=w71:path)
      n153 = Create Folder(path (use dialog)=w78) -> (created path=w82:path)  [unwired: 2 in, 2 out]
      n154 = Create Folder(path (use dialog)=w130) -> (created path=w129:path)  [unwired: 2 in, 2 out]
      n155 = Create Folder(path (use dialog)=w132) -> (created path=w131:path)  [unwired: 2 in, 2 out]
      n156 = Copy(10:w71, 11:w81) -> ()  [unwired: 3 in, 3 out]
      n157 = Strip Path(path=w77) -> (name=w79:string)  [unwired: 1 out]
      n158 = case shown="True" w147 {
        tunnel: [w302 w307] -> w251
        tunnel: [w302 w306] -> w250
        tunnel: w82 -> [_ w305]
        tunnel: w209 -> [_ w304]
        tunnel: w145 -> [_ w303]
        frame False {
          w302 = refnum<k34> refnum ("tdms1")
        }
        frame True {
          n159 = call "TDMS0.vi"("Startmethode"=w303, "Dateiname"=w304, "Dateiordner"=w305) -> ("tdms1"=w306:refnum<k34>, "tdms0"=w307:refnum<k34>)
          n160 = global write "GVaktuelleTDMS.vi" "aktuelleTDMS-DateiHK"(w307) -> ()
        }
      }
      n161 = case shown="True" w147 {
        tunnel: [w292 w301] -> w249
        tunnel: [w292 w300] -> w248
        tunnel: [w292 w299] -> w247
        tunnel: [w292 w298] -> w246
        tunnel: w129 -> [_ w297]
        tunnel: w208 -> [_ w296]
        tunnel: w131 -> [_ w295]
        tunnel: w207 -> [_ w294]
        tunnel: w145 -> [_ w293]
        frame False {
          w292 = refnum<k34> refnum ("tdms0")
        }
        frame True {
          n162 = call "TDMS0.vi"("Startmethode"=w293, "Dateiname"=w296, "Dateiordner"=w297) -> ("tdms1"=w300:refnum<k34>, "tdms0"=w301:refnum<k34>)
          n163 = call "TDMS0.vi"("Startmethode"=w293, "Dateiname"=w294, "Dateiordner"=w295) -> ("tdms1"=w298:refnum<k34>, "tdms0"=w299:refnum<k34>)
          n164 = global write "GVaktuelleTDMS.vi" "aktuelleTDMS-DateiECD1"(w301) -> ()
          n165 = global write "GVaktuelleTDMS.vi" "aktuelleTDMS-DateiECD2"(w299) -> ()
        }
      }
      n166 = Build Path(base path=w69, name or relative path=w79) -> (appended path=w70:path)
      n167 = Copy(10:w70, 11:w77) -> ()  [unwired: 3 in, 3 out]
      n168 = Open/Create/Replace File(file path (use dialog)=path "c:/fromcriocmd.txt" ("Pfad MS-Datei CRIO"), operation (0:open)=T13."replace or create" ("Operation (0:Öffnen)")) -> (refnum out=w243:refnum<file>, error out=w242:errorcluster)  [unwired: 4 in, 1 out]
      n169 = Write to Text File(file (use dialog)=w243, text="time=yyyymmddhhmmss\ncycle=005\ninfo=1234567890123456789012345678901234567890123456789012345678901234567890123456789012345678901234567890\nlength=100\ncmd=cycle" ("Text0 MS-Datei"), error in=w242) -> (refnum out=w240:refnum<file>, error out=w239:errorcluster)  [unwired: 1 in, 1 out]
      n170 = Bundle("created path"=w82, "created path"=w129, "created path"=w131, "Dateiname Housekeeping"=w209, "DateinameECD1"=w208, "DateinameECD2"=w207, "tdms0"=w251, "tdms1"=w250, "tdms0"=w249, "tdms1"=w248, "tdms0"=w247, "tdms1"=w246) -> (w252:T19)  [unwired: 1 in]
      n171 = call "AIKoeffSortieren.vi"("Modul3/AI koeff"=w214, "Modul2/AI koeff"=w215, "Modul1/AI koeff"=w216) -> ("P0"=w255:dbl[], "P1"=w256:dbl[], "P2"=w257:dbl[])
      n172 = Close File(refnum=w240, error in=w239) -> (path=w234:path)  [unwired: 1 out]
      "schnelle Heizungen" <- w76
    }
    frame #1 {
      w322 = dbl[] [-1.0]
      w393 = 0
      w368 = 0 ("Zyklusnummer1")
      n173 = Add Array Elements(numeric array=w342) -> (sum=w341:i32)
      n174 = Array Size(array=w350) -> (size(s)=w371:i32)
      n175 = Unbundle(w367) -> ("created path"=w366:path, "created path"=w364:path, "created path"=w363:path, "Dateiname Housekeeping"=w365:string, "DateinameECD1"=w362:string, "DateinameECD2"=w361:string, "tdms0"=w360:refnum<k34>, "tdms1"=w359:refnum<k34>, "tdms0"=w358:refnum<k34>, "tdms1"=w357:refnum<k34>, "tdms0"=w356:refnum<k34>, "tdms1"=w355:refnum<k34>)
      n176 = Index Array(array=w343, index #1=0 ("Index"), index #2=1 ("Index"), index #3=2 ("Index"), index #4=3 ("Index")) -> (element #1=w382:i32, element #2=w381:i32, element #3=w384:i32, element #4=w383:i32)
      n177 = flat-sequence {
        frame #0 {
          n178 = global write "Emulate Licor output GV.vi" "Emulator an?"(FALSE ("Emulator an?")) -> ()
        }
        frame #1 {
          n179 = control-ref of="GUI_Cluster_sdv"() -> (w421:refnum<vi>)
          n180 = control-ref of="GUI_Cluster_Graph"() -> (w423:refnum<vi>)
          n181 = control-ref of="GUI_Cluster_Parameter"() -> (w422:refnum<vi>)
          n182 = call "licore (main).vi"("GUI_Cluster_Graph (extern)"=w423, "GUI_Cluster_Parameter (extern)"=w422, "GUI_Cluster_sdv (extern)"=w421) -> ()  [unwired: 13 in]
        }
      }
      n183 = while {
        shift-right: ["Methode"] -> _
        shift-left: w419 -> [w1210]
        stop <- w1212 stop-if-true
        n184 = call "Bis zum nächsten Vielfachen warten7"("Count(mSec)"=u32 1000) -> ()  [unwired: 1 out]
        n185 = Not Equal?(x=w1210, y="Methode") -> (x != y?=w1208:bool)
        n186 = global read "gvbooleschRT.vi" "global stop RT"() -> (w1212:bool)
        n187 = global write "GVMethodenwechsel.vi" "Methodenwechsel?"(w1208) -> ()
      }
      n188 = call <vilib>:"Space Constant.vi"() -> ("String"=w328:string)
      n189 = while {
        tunnel: w346 -> [w657]
        tunnel: w415 -> [w660]
        tunnel: w414 -> [w659]
        tunnel: w413 -> [w658]
        shift-right: [w662] -> _
        shift-left: errorcluster {"status"=FALSE, "code"=0, "source"=""} ("error out") -> [w661]
        stop <- w663 stop-if-true
        n190 = call "AIsFIFORT-15-07-17.vi"("FPGA VI Reference In"=w657, "P2"=w660, "P1"=w659, "P0"=w658, "error in"=w661) -> ("error out"=w662:errorcluster)
        "AIsFIFOread" <- w662
        n191 = global read "gvbooleschRT.vi" "global stop RT"() -> (w663:bool)
      }
      n192 = while {
        tunnel: w346 -> [w664]
        tunnel: w321 -> [w667]
        tunnel: w320 -> [w666]
        tunnel: w319 -> [w665]
        shift-right: [w669] -> _
        shift-left: errorcluster {"status"=FALSE, "code"=0, "source"=""} ("error out") -> [w668]
        stop <- w671 stop-if-true
        n193 = call "Bis zum nächsten Vielfachen warten16"("Count(mSec)"=u32 100) -> ()  [unwired: 1 out]
        n194 = call "TrapsMachMitteln-15-07-17.vi"("FPGA VI Reference In"=w664, "Traps/MachKoeff2"=w667, "Traps/MachKoeff1"=w666, "Traps/MachKoeff0"=w665, "error in"=w668) -> ("error out"=w669:errorcluster)
        "MWTrapsMachs" <- w669
        n195 = global read "gvbooleschRT.vi" "global stop RT"() -> (w671:bool)
      }
      n196 = for {
        N: 1 -> [_]
        tunnel: w346 -> [w672]
        tunnel: [w672] -> w373
        n197 = call "Warten8"("Count(mSec)"=u32 100) -> ()  [unwired: 1 out]
      }
      n198 = Build Array(w328) -> (w327:string[])
      n199 = Initialize Array(-1 ("Element"), 4 ("Dimension")) -> (w344:i32[])
      n200 = global read "GVVentilposition.vi" "Ventilposition"() -> (w352:i32)
      n201 = Add(x=w384, y=w383) -> (x+y=w380:i32)
      n202 = Bundle(w327, w327, w327) -> (w391:cluster{string[], string[], string[]})  [unwired: 1 in]
      n203 = Index Array(array=w337, index=w335) -> (element=w336:T16)
      n204 = Initialize Array(cluster{"output high":dbl, "output low":dbl} {"output high"=99999.0, "output low"=0.0} ("output range"), w371) -> (w351:cluster{"output high":dbl, "output low":dbl}[])
      n205 = while {
        tunnel: w418 -> [w788]
        shift-right: [w787] -> _
        shift-left: w337 -> [w769]
        tunnel: w351 -> [w786]
        tunnel: w350 -> [w785]
        tunnel: w346 -> [w784]
        tunnel: w349 -> [w783]
        tunnel: w348 -> [w782]
        shift-right: [w776] -> _
        shift-left: 0 -> [w781]
        tunnel: w346 -> [w780]
        tunnel: w345 -> [w779]
        shift-right: [w775] -> _
        shift-left: w344 -> [w778]
        tunnel: w343 -> [w770]
        tunnel: w342 -> [w771]
        tunnel: w341 -> [w772]
        tunnel: w340 -> [w773]
        tunnel: w339 -> [w774]
        tunnel: w338 -> [w777]
        shift-right: [w693] -> _
        shift-left: w336 -> [w692]
        tunnel: w321 -> [w678]
        tunnel: w320 -> [w679]
        tunnel: w319 -> [w680]
        tunnel: w314 -> [w681]
        tunnel: w313 -> [w677]
        i -> [w696]
        stop <- w789 stop-if-true
        w686 = 0  # ZeileMainMach2
        w687 = 0  # ZeileMainMach1
        w737 = FALSE
        w736 = 0.0
        w738 = 0  # ZeilennummerMPV
        w742 = cluster{dbl[], dbl[]} {[], []}
        w751 = dbl[] []
        w755 = 0  # ZeilePreMach2
        w756 = 0  # ZeilePreMach1
        w757 = 0  # ZeileFPGAFixp
        w758 = 0  # ZeileFPGAPID
        w759 = 0  # ZeileFPGABoolesch
        w760 = i32[] [0, 0, 0, 0]  # ZeilennummernHorst
        w761 = i32[] [0, 0, 0, 0]  # ZeilennummernDIOs
        n206 = Unbundle(w677) -> ("created path"=w676:path, "created path"=w675:path)
        n207 = Unbundle(w692) -> ("Zykluslängen [s]"=w674:dbl[], "ZeitpktDIOsMod0"=w735:dbl[], "ZeitpktDIOsMod1"=w734:dbl[], "ZeitpktDIOsMod2A"=w733:dbl[], "ZeitpktDIOsMod2B"=w732:dbl[], "DIOsSPMod0"=w731:bool[][], "DIOsSPMod1"=w730:bool[][], "DIOsSPMod2A"=w729:bool[][], "DIOsSPMod2B"=w728:bool[][], "Mod0HorstZeitpkt"=w727:dbl[], "Mod1HorstZeitpkt"=w726:dbl[], "Mod2AHorstZeitpkt"=w725:dbl[], "Mod2BHorstZeitpkt"=w724:dbl[], "HorstSPMod0"=w723:dbl[][], "HorstSPMod1"=w722:dbl[][], "HorstSPMod2A"=w721:dbl[][], "HorstSPMod2B"=w720:dbl[][], "LHSetpoints"=w719:dbl[], "LHHeizen?"=w718:bool[], "ZPktFPGABoolesch"=w717:dbl[], "FPGABoolesch"=w716:bool[][], "ZeitpktFPGAPID"=w715:dbl[], "FPGAPID"=w714:T20, "ZeitpktFPGAFixp"=w713:dbl[], w712:dbl[][], "t_PreMach1"=w711:dbl[], "T_PreMach1"=w710:dbl[], "t_PreMach2"=w709:dbl[], "T_PreMach2"=w708:dbl[], "PIDs für \"träge\" Heizungen"=w707:T21, "Zwangsbedingungen"=w706:dbl[][], "Dateien fürs MS schicken?"=w705:bool, "ZeitpunkteMPV"=w704:dbl[], "SPMPV"=w703:i32[], "ZeitpktMS-1"=w702:dbl, "ZeitpktMS-2"=w701:dbl, "Int.Start1"=w700:dbl, "Int.Stop1"=w699:dbl, "Int.Start2"=w698:dbl, "Int.Stop2"=w697:dbl, "t_MainMach1"=w691:dbl[], "T_MainMach1"=w690:dbl[], "t_MainMach2"=w689:dbl[], "T_MainMach2"=w688:dbl[])  [unwired: 1 out]
        n208 = while {
          tunnel: w674 -> [w822]
          tunnel: w675 -> [w812]
          stop <- w811 stop-if-true
          n209 = global read "GVZeitenZyklen.vi" "Big Ben, Methodenzeit, Zykluszeit0, Zykluszeit1, Zykluszeit2A, Zykluszeit2B"() -> (w820:dbl[])
          n210 = Index Array(array=w820, index=5) -> (element=w818:dbl)
          n211 = global read "GVZeitenZyklen.vi" "ZyklusNummernGesamt"() -> (w823:i32[])
          n212 = call "Wait Until Next Multiple2"("Count(mSec)"=u32 100) -> ()  [unwired: 1 out]
          n213 = Index Array(array=w822, index=3) -> (element=w817:dbl)
          n214 = Subtract(x=w817, y=0.2) -> (x-y=w815:dbl)
          n215 = Greater Or Equal?(x=w818, y=w815) -> (x >= y?=w814:bool)
          n216 = global read "GVChroms.vi" "ECD2Chrom"() -> (w813:dbl[])
          n217 = case shown="True" w814 {
            tunnel: w823 -> [_ w831]
            tunnel: w813 -> [_ w830]
            tunnel: w812 -> [_ w829]
            frame False {
            }
            frame True {
              n218 = flat-sequence {
                tunnel: w831 -> [w847]
                tunnel: w830 -> [w834]
                tunnel: w829 -> [w833]
                frame #0 {
                  n219 = Index Array(array=w847, index=3) -> (element=w845:i32)
                  n220 = Number To Decimal String(number=w845, width (-)=i16 4) -> (decimal integer string=w843:string)
                  n221 = Concatenate Strings(w843, "ECD2.hag" ("string")) -> (w841:string)
                  n222 = Build Path(base path=w833, name or relative path=w841) -> (appended path=w832:path)
                  n223 = Open/Create/Replace File(file path (use dialog)=w832, operation (0:open)=T13."replace or create") -> (refnum out=w840:refnum<file>, error out=w839:errorcluster)  [unwired: 4 in, 1 out]
                  n224 = Write to Binary File(file (use dialog)=w840, data=w834, error in=w839) -> (refnum out=w838:refnum<file>, error out=w837:errorcluster)  [unwired: 3 in, 1 out]
                  n225 = Close File(refnum=w838, error in=w837) -> (error out=→"ECD2dataBackup":errorcluster)  [unwired: 1 out]
                }
                frame #1 {
                  n226 = call "Wait2"("Count(mSec)"=u32 2000) -> ()  [unwired: 1 out]
                }
              }
            }
          }
          n227 = global read "GVMethodenwechsel.vi" "Methodenwechsel?"() -> (w826:bool)
          n228 = global read "gvbooleschRT.vi" "global stop RT"() -> (w827:bool)
          n229 = Or(x=w826, y=w827) -> (x .or. y?=w828:bool)
          n230 = local read "veränderte Methode benutzen"() -> (w825:bool)
          n231 = Or(x=w828, y=w825) -> (x .or. y?=w811:bool)
        }
        n232 = while {
          tunnel: w674 -> [w859]
          tunnel: w676 -> [w849]
          stop <- w863 stop-if-true
          n233 = global read "GVZeitenZyklen.vi" "Big Ben, Methodenzeit, Zykluszeit0, Zykluszeit1, Zykluszeit2A, Zykluszeit2B"() -> (w857:dbl[])
          n234 = Index Array(array=w857, index=4) -> (element=w855:dbl)
          n235 = global read "GVZeitenZyklen.vi" "ZyklusNummernGesamt"() -> (w860:i32[])
          n236 = call "Wait Until Next Multiple"("Count(mSec)"=u32 100) -> ()  [unwired: 1 out]
          n237 = Index Array(array=w859, index=2) -> (element=w854:dbl)
          n238 = Subtract(x=w854, y=0.2) -> (x-y=w852:dbl)
          n239 = Greater Or Equal?(x=w855, y=w852) -> (x >= y?=w851:bool)
          n240 = global read "GVChroms.vi" "ECD1Chrom"() -> (w850:dbl[])
          n241 = case shown="True" w851 {
            tunnel: w860 -> [_ w869]
            tunnel: w850 -> [_ w868]
            tunnel: w849 -> [_ w867]
            frame False {
            }
            frame True {
              n242 = flat-sequence {
                tunnel: w869 -> [w885]
                tunnel: w868 -> [w872]
                tunnel: w867 -> [w871]
                frame #0 {
                  n243 = Index Array(array=w885, index=2) -> (element=w883:i32)
                  n244 = Number To Decimal String(number=w883, width (-)=i16 4) -> (decimal integer string=w881:string)
                  n245 = Concatenate Strings(w881, "ECD1.hag" ("string")) -> (w879:string)
                  n246 = Build Path(base path=w871, name or relative path=w879) -> (appended path=w870:path)
                  n247 = Open/Create/Replace File(file path (use dialog)=w870, operation (0:open)=T13."replace or create") -> (refnum out=w878:refnum<file>, error out=w877:errorcluster)  [unwired: 4 in, 1 out]
                  n248 = Write to Binary File(file (use dialog)=w878, data=w872, error in=w877) -> (refnum out=w876:refnum<file>, error out=w875:errorcluster)  [unwired: 3 in, 1 out]
                  n249 = Close File(refnum=w876, error in=w875) -> (error out=→"ECD1dataBackup":errorcluster)  [unwired: 1 out]
                }
                frame #1 {
                  n250 = call "Wait"("Count(mSec)"=u32 2000) -> ()  [unwired: 1 out]
                }
              }
            }
          }
          n251 = global read "GVMethodenwechsel.vi" "Methodenwechsel?"() -> (w864:bool)
          n252 = global read "gvbooleschRT.vi" "global stop RT"() -> (w865:bool)
          n253 = Or(x=w864, y=w865) -> (x .or. y?=w866:bool)
          n254 = local read "veränderte Methode benutzen"() -> (w862:bool)
          n255 = Or(x=w866, y=w862) -> (x .or. y?=w863:bool)
        }
        n256 = Add(x=w778, y=1) -> (x+y=w746:i32[])
        n257 = local read "Methode"() -> (w695:i32)
        n258 = Build Cluster Array(w731, w730, w729, w728) -> (w765:cluster{"DIOsSPMod2B":bool[][]}[])
        n259 = Build Cluster Array(w723, w722, w721, w720) -> (w763:cluster{"HorstSPMod2B":dbl[][]}[])
        n260 = Build Cluster Array(w735, w734, w733, w732) -> (w766:cluster{"ZeitpktDIOsMod2B":dbl[]}[])
        n261 = Build Cluster Array(w727, w726, w725, w724) -> (w764:cluster{"Mod2BHorstZeitpkt":dbl[]}[])
        n262 = Equal?(x=w696, y=0) -> (x = y?=w767:bool)
        n263 = while {
          tunnel: w674 -> [w797]
          stop <- w800 stop-if-true
          n264 = global read "GVZeitenZyklen.vi" "Big Ben, Methodenzeit, Zykluszeit0, Zykluszeit1, Zykluszeit2A, Zykluszeit2B"() -> (w806:dbl[])
          n265 = To Long Integer(number="Zyklus") -> (32bit integer=w792:i32)
          n266 = Index Array(array=w797, index=w792) -> (element=w796:dbl)
          n267 = Subtract(x=w796, y=1.0) -> (x-y=w794:dbl)
          n268 = Add(x=w792, y=2) -> (x+y=w790:i32)
          n269 = call "Wait3"("Count(mSec)"=u32 100) -> ()  [unwired: 1 out]
          n270 = global read "GVMethodenwechsel.vi" "Methodenwechsel?"() -> (w802:bool)
          n271 = global read "gvbooleschRT.vi" "global stop RT"() -> (w803:bool)
          n272 = local read "am Ende benutzen"() -> (w805:bool)
          n273 = local read "veränderte Methode benutzen"() -> (w798:bool)
          n274 = Index Array(array=w806, index=w790) -> (element=w807:dbl)
          n275 = Or(x=w802, y=w803) -> (x .or. y?=w801:bool)
          n276 = Greater Or Equal?(x=w807, y=w794) -> (x >= y?=w808:bool)
          n277 = And(x=w808, y=w805) -> (x .and. y?=w799:bool)
          n278 = case shown="True" w799 {
            frame False {
            }
            frame True {
              n279 = local write "veränderte Methode benutzen"(TRUE ("veränderte Methode benutzen")) -> ()
              n280 = local write "am Ende benutzen"(FALSE ("am Ende benutzen")) -> ()
            }
          }
          n281 = Or(x=w801, y=w798) -> (x .or. y?=w800:bool)
        }
        n282 = while {
          tunnel: w771 -> [w955]
          tunnel: w774 -> [w948]
          tunnel: w773 -> [w949]
          tunnel: w770 -> [w954]
          tunnel: w772 -> [w950]
          tunnel: w706 -> [w951]
          stop <- w957 stop-if-true
          n283 = call "Bis zum nächsten Vielfachen warten10"("Count(mSec)"=u32 1000) -> ()  [unwired: 1 out]
          n284 = local read "Methode"() -> (w953:i32)
          n285 = global read "GVMethodenwechsel.vi" "Methodenwechsel?"() -> (w959:bool)
          n286 = global read "gvbooleschRT.vi" "global stop RT"() -> (w960:bool)
          n287 = case shown="True" "global stop RT" {
            frame False {
            }
            frame True {
              n288 = global write "gvbooleschRT.vi" "global stop RT"(TRUE ("global stop RT")) -> ()
            }
          }
          n289 = call "ZwangsbedingungenGV-15-07-17.vi"("AnzahlHorst"=w948, "AnzahlHorst/Modul"=w954, "AnzahlLH"=w949, "AnzahlDIOs/Modul"=w955, "AnzahlDIOs"=w950, "Zwangsbedingungen"=w951, "Methodennummer"=w953) -> ("Methodennummer"=w952:i32)  [unwired: 4 in]
          n290 = local write "Methode"(w952) -> ()
          n291 = local read "veränderte Methode benutzen"() -> (w958:bool)
          n292 = Compound Arithmetic op=OR(w960, w959, w958) -> (w957:bool)
        }
        n293 = global read "GVZeitenZyklen.vi" "ZyklusNummern"() -> (w745:i32[])
        n294 = global read "GVZwangs.vi" "ZwangsHorst?"() -> (w750:cluster{bool[]}[])
        n295 = global read "gvbooleschRT.vi" "global stop RT"() -> (w789:bool)
        n296 = global read "GVZwangsMPV.vi" "ZwangsMPV?"() -> (w684:bool)
        n297 = global read "GVZwangs.vi" "ZwangsDIO?"() -> (w749:cluster{bool[]}[])
        n298 = global read "GVaktuelleTDMS.vi" "aktuelleTDMS-DateiECD1"() -> (w744:refnum<k34>)
        n299 = Bundle(w766, w765, w764, w763, "LHHeizen?"=w718, "ZPktFPGABoolesch"=w717, "FPGABoolesch"=w716, "ZeitpktFPGAPID"=w715, "FPGAPID"=w714, "ZeitpktFPGAFixp"=w713, w712, "t_PreMach1"=w711, "T_PreMach1"=w710, "t_PreMach2"=w709, "T_PreMach2"=w708, "ZeitpunkteMPV"=w704, "SPMPV"=w703, "t_MainMach1"=w691, "T_MainMach1"=w690, "t_MainMach2"=w689, "T_MainMach2"=w688) -> (w762:T22)  [unwired: 1 in]
        n300 = Index Array(array=w769, index=w695) -> (element=w694:T16)
        n301 = global read "GVZwangs.vi" "ZwangsFPGABoolesch?"() -> (w748:bool[])
        n302 = while {
          tunnel: w785 -> [w938]
          tunnel: w786 -> [w941]
          tunnel: w784 -> [w942]
          tunnel: w719 -> [w939]
          tunnel: w707 -> [w940]
          shift-right: [w936] -> _
          shift-left: errorcluster {"status"=FALSE, "code"=0, "source"=""} ("error out") -> [w937]
          stop <- w943 stop-if-true
          n303 = call "LH-15-07-17.vi"("FPGA VI Reference In"=w942, "OutputRange"=w941, "LHSetpoints"=w939, "AIsLH"=w938, "error in"=w937, "LH-Gruppe"="LH-Gruppe", "PIDs für \"träge\" Heizungen"=w940) -> ("error out"=w936:errorcluster)
          "LH" <- w936
          n304 = call "Bis zum nächsten Vielfachen warten12"("Count(mSec)"=u32 100) -> ()  [unwired: 1 out]
          n305 = global read "GVMethodenwechsel.vi" "Methodenwechsel?"() -> (w945:bool)
          n306 = global read "gvbooleschRT.vi" "global stop RT"() -> (w946:bool)
          n307 = local read "veränderte Methode benutzen"() -> (w944:bool)
          n308 = Compound Arithmetic op=OR(w946, w945, w944) -> (w943:bool)
        }
        n309 = while {
          shift-right: [w899] -> _
          shift-left: w737 -> [w903]
          shift-right: [w898] -> _
          shift-left: w736 -> [w902]
          shift-right: [w897] -> _
          shift-left: w737 -> [w901]
          shift-right: [w896] -> _
          shift-left: w736 -> [w900]
          tunnel: w777 -> [w895]
          tunnel: w700 -> [w890]
          tunnel: w699 -> [w889]
          tunnel: w698 -> [w888]
          tunnel: w697 -> [w887]
          stop <- w892 stop-if-true
          n310 = call "Integrieren.vi"("Integrieren1"=w903, "Integral1"=w902, "Integrieren2"=w901, "Integral2"=w900, "Int.Start1"=w890, "Int.Stop1"=w889, "Int.Start2"=w888, "HorstProbenflußNr."=w895, "Int.Stop2"=w887) -> ("Integrieren1"=w899:bool, "Integral1"=w898:dbl, "Integrieren2"=w897:bool, "Integral2"=w896:dbl)  [unwired: 7 in]
          n311 = call "Bis zum nächsten Vielfachen warten9"("Count(mSec)"=u32 100) -> ()  [unwired: 1 out]
          n312 = global read "GVMethodenwechsel.vi" "Methodenwechsel?"() -> (w893:bool)
          n313 = global read "gvbooleschRT.vi" "global stop RT"() -> (w894:bool)
          n314 = local read "veränderte Methode benutzen"() -> (w891:bool)
          n315 = Compound Arithmetic op=OR(w894, w893, w891) -> (w892:bool)
        }
        n316 = while "Zeit" {
          tunnel: w767 -> [w1147]
          tunnel: w674 -> [w1145]
          tunnel: w746 -> [w1140]
          tunnel: [w1139] -> w775
          shift-right: [w1136] -> _
          shift-left: 0.0 -> [w1137]
          i -> [w1149]
          stop <- w1142 stop-if-true
          n317 = Equal?(x=w1149, y=0) -> (x = y?=w1138:bool)
          n318 = call "Bis zum nächsten Vielfachen warten15"("Count(mSec)"=u32 50) -> ()  [unwired: 1 out]
          n319 = call "BigBen-01-16.vi"("MethodenStartzeit"=w1137, "Methodenstart?"=w1138, "Programmstart?"=w1147, "Zykluslängen [s]"=w1145, "MethodenStartZyklusNummern"=w1140) -> ("MethodenStartzeit"=w1136:dbl, "ZyklusNummernGesamt"=w1139:i32[])  [unwired: 2 in]
          n320 = global read "GVMethodenwechsel.vi" "Methodenwechsel?"() -> (w1141:bool)
          n321 = global read "gvbooleschRT.vi" "global stop RT"() -> (w1146:bool)
          n322 = Or(x=w1141, y=w1146) -> (x .or. y?=w1143:bool)
          n323 = local read "veränderte Methode benutzen"() -> (w1144:bool)
          n324 = Or(x=w1144, y=w1143) -> (x .or. y?=w1142:bool)
        }
        n325 = Bundle(w751, w751, w751, w751) -> (w752:cluster{dbl[], dbl[], dbl[], dbl[]})  [unwired: 1 in]
        n326 = while {
          tunnel: w788 -> [w1162]
          shift-right: [w1153] -> _
          shift-left: w694 -> [w1161]
          tunnel: w695 -> [w1159]
          shift-right: [w1151] -> w787
          shift-left: w769 -> [w1160]
          tunnel: [w1152] -> w693
          stop <- w1155 stop-if-true
          n327 = call "Bis zum nächsten Vielfachen warten8"("Count(mSec)"=u32 500) -> ()  [unwired: 1 out]
          n328 = global read "GVMethodenwechsel.vi" "Methodenwechsel?"() -> (w1157:bool)
          n329 = global read "gvbooleschRT.vi" "global stop RT"() -> (w1156:bool)
          n330 = case shown="True" "Methode verändern" {
            tunnel: w1162 -> [_ w1184]
            tunnel: w1161 -> [w1181 w1183]
            tunnel: [w1181 w1182] -> w1153
            frame False {
            }
            frame True {
              n331 = call "methodeändern-15-07-17.vi"("->Methode"=w1183, "Namen"=w1184) -> ("Methode->"=w1182:T23)  [unwired: 1 in]
              n332 = property on="Methode verändern" class="Bool. (strikt)"("Value"=FALSE ("Methode verändern")) -> ()  [unwired: 2 in, 2 out]
            }
          }
          n333 = Compound Arithmetic op=OR(w1157, w1156, "veränderte Methode benutzen") -> (w1155:bool)
          n334 = case shown="True" "Methode speichern" {
            tunnel: w1153 -> [_ w1178]
            tunnel: w1160 -> [w1171 w1180]
            tunnel: w1159 -> [_ w1179]
            tunnel: [w1171 w1173] -> w1151
            frame False {
            }
            frame True {
              n335 = Replace Array Subset(array=w1180, new element=w1178, index=w1179) -> (w1173:T11)
              n336 = property on="Methode speichern" class="Bool. (strikt)"("Value"=FALSE ("Methode speichern")) -> ()  [unwired: 2 in, 2 out]
              n337 = Open/Create/Replace File(file path (use dialog)=path "c:/methoden.pery" ("Dateipfad (Dialog verwenden)"), operation (0:open)=T13."replace" ("Operation (0:Öffnen)")) -> (refnum out=w1175:refnum<file>)  [unwired: 4 in, 2 out]
              n338 = Write to Binary File(file (use dialog)=w1175, data=w1173) -> (refnum out=w1172:refnum<file>)  [unwired: 4 in, 2 out]
              n339 = Close File(refnum=w1172) -> ()  [unwired: 1 in, 2 out]
            }
          }
          n340 = case shown="True" "veränderte Methode benutzen" {
            tunnel: w1153 -> [_ w1168]
            tunnel: [w1165 w1168] -> w1152
            tunnel: w1151 -> [w1167 _]
            frame False {
              n341 = local read "Methode"() -> (w1166:i32)
              n342 = Index Array(array=w1167, index=w1166) -> (element=w1165:T16)
            }
            frame True {
              n343 = flat-sequence {
                frame #0 {
                  n344 = call "Warten"("Count(mSec)"=u32 1100) -> ()  [unwired: 1 out]
                }
                frame #1 {
                  n345 = property on="veränderte Methode benutzen" class="Bool. (strikt)"("Value"=FALSE ("Methode verändern")) -> ()  [unwired: 2 in, 2 out]
                }
              }
            }
          }
        }
        n346 = Bundle("ZyklusNummern"=w745, "ZeilennummernDIOs"=w761, "ZwangsDIO?"=w749, "ZeilennummernHorst"=w760, "ZwangsHorst?"=w750, "ZeileFPGABoolesch"=w759, "ZwangsFPGABoolesch?"=w748, "ZeileFPGAPID"=w758, "ZeileFPGAFixp"=w757, "ZeilePreMach1"=w756, "ZeilePreMach2"=w755, "ZeilennummerMPV"=w738, "ZeileMainMach1"=w687, "ZeileMainMach2"=w686, "ZwangsMPV?"=w684) -> (w754:T24)  [unwired: 1 in]
        n347 = while {
          shift-right: [w1079] -> _
          shift-left: w752 -> [w1086]
          shift-right: [w1078] -> _
          shift-left: w752 -> [w1085]
          shift-right: [w1076] -> _
          shift-left: T14 {"Zyklus1"=0, "Zeitachse1"=0, "dargestellte Größe 1"=0, "Zyklus2"=0, "Zeitachse2"=0, "dargestellte Größe 2"=0} ("AnzeigeEinstellungen") -> [w1084]
          tunnel: w674 -> [w1054]
          shift-right: [w1050] -> _
          shift-left: w744 -> [w1049]
          shift-right: [w1045] -> _
          shift-left: w742 -> [w1047]
          shift-right: [w1034] -> _
          shift-left: w742 -> [w1046]
          shift-right: ["Detektor"] -> _
          shift-left: 0 ("Detektor") -> [w1043]
          tunnel: w681 -> [w1032]
          stop <- w1090 stop-if-true
          w1055 = 0.0 ("X-Achse.Bereich:Minimum")
          n348 = Unbundle(w1032) -> ("Modul1/AI sicherer Bereich"=w1025:dbl[][], "Modul2/AI sicherer Bereich"=w1010:dbl[][], "Modul3/AI sicherer Bereich"=w1001:dbl[][], "Traps/Machs sicherer Bereich"=w992:dbl[][], w984:dbl[][], "Metavariablen grüner Bereich"=w975:dbl[][])
          n349 = call "Bis zum nächsten Vielfachen warten14"("Count(mSec)"=u32 1000) -> ()  [unwired: 1 out]
          n350 = global read "GVMWHorst.vi" "MWHorst"() -> (w983:dbl[])
          "MWHorst" <- w983
          n351 = case shown="0, Standard" "Detektor" {
            tunnel: [w1100 w1112] -> w1045
            tunnel: w1054 -> [w1099 w1114]
            tunnel: "Detektor" -> [w1094 w1108]
            tunnel: [w1098 w1113] -> w1052
            tunnel: [w1097 w1111] -> w1050
            frame 0, Default {
              n352 = Increment(x=w1094) -> (x+1=w1095:i32)
              n353 = Increment(x=w1095) -> (x+1=w1093:i32)
              n354 = global read "GVChroms.vi" "ECD1Chrom"() -> (w1096:dbl[])
              n355 = global read "GVaktuelleTDMS.vi" "aktuelleTDMS-DateiECD1"() -> (w1097:refnum<k34>)
              n356 = Index Array(array=w1099, index=w1093) -> (element=w1098:dbl)
              n357 = Array Size(array=w1096) -> (size(s)=w1102:i32)
              n358 = for {
                N: w1102 -> [_]
                tunnel: [w1103] -> w1101 mode=indexing
                i -> [w1106]
                n359 = To Double Precision Float(number=w1106) -> (double precision float=w1105:dbl)
                n360 = Divide(x=w1105, y=10.0) -> (x/y=w1103:dbl)
              }
              n361 = Bundle(w1101, "ECD1Chrom"=w1096) -> (w1100:cluster{dbl[], "ECD1Chrom":dbl[]})  [unwired: 1 in]
            }
            frame 1 {
              n362 = Increment(x=w1108) -> (x+1=w1109:i32)
              n363 = Increment(x=w1109) -> (x+1=w1107:i32)
              n364 = global read "GVChroms.vi" "ECD2Chrom"() -> (w1110:dbl[])
              n365 = global read "GVaktuelleTDMS.vi" "aktuelleTDMS-DateiECD2"() -> (w1111:refnum<k34>)
              n366 = Index Array(array=w1114, index=w1107) -> (element=w1113:dbl)
              n367 = Array Size(array=w1110) -> (size(s)=w1116:i32)
              n368 = for {
                N: w1116 -> [_]
                tunnel: [w1117] -> w1115 mode=indexing
                i -> [w1120]
                n369 = To Double Precision Float(number=w1120) -> (double precision float=w1119:dbl)
                n370 = Divide(x=w1119, y=10.0) -> (x/y=w1117:dbl)
              }
              n371 = Bundle(w1115, "ECD2Chrom"=w1110) -> (w1112:cluster{dbl[], "ECD2Chrom":dbl[]})  [unwired: 1 in]
            }
          }
          n372 = Subtract(x="DetYMax", y="DetYMin") -> (x-y=w1060:dbl)
          n373 = Subtract(x="HK1YMax", y="HK1YMin") -> (x-y=w1070:dbl)
          n374 = Subtract(x="HK2YMax", y="HK2YMin") -> (x-y=w1065:dbl)
          n375 = Equal?(x="Detektor", y=w1043) -> (x = y?=w1042:bool)
          n376 = Index Array(array=w1025, index (col) #1=0 ("disabled index (col)"), index (col) #2=1 ("index (col)")) -> (element #1=w1022:dbl[], element #2=w1020:dbl[])  [unwired: 2 in]
          n377 = Index Array(array=w1010, index (col) #1=0 ("disabled index (col)"), index (col) #2=1 ("index (col)")) -> (element #1=w1014:dbl[], element #2=w1013:dbl[])  [unwired: 2 in]
          n378 = Index Array(array=w992, index (col) #1=0 ("disabled index (col)"), index (col) #2=1 ("index (col)")) -> (element #1=w996:dbl[], element #2=w995:dbl[])  [unwired: 2 in]
          n379 = Index Array(array=w984, index (col) #1=0 ("disabled index (col)"), index (col) #2=1 ("index (col)")) -> (element #1=w988:dbl[], element #2=w987:dbl[])  [unwired: 2 in]
          n380 = Index Array(array=w1001, index (col) #1=0 ("disabled index (col)"), index (col) #2=1 ("index (col)")) -> (element #1=w1005:dbl[], element #2=w1004:dbl[])  [unwired: 2 in]
          n381 = Index Array(array=w975, index (col) #1=0 ("disabled index (col)"), index (col) #2=1 ("index (col)")) -> (element #1=w979:dbl[], element #2=w978:dbl[])  [unwired: 2 in]
          n382 = global read "GVMethodenwechsel.vi" "Methodenwechsel?"() -> (w1088:bool)
          n383 = global read "GVZeitenZyklen.vi" "ZyklusNummern"() -> (w1057:i32[])
          "ZyklusNummern" <- w1057
          n384 = global read "gvbooleschRT.vi" "global stop RT"() -> (w1089:bool)
          n385 = global read "GVMetavariablen.vi" "Metavariablen"() -> (w974:dbl[])
          "MVWerte" <- w974
          n386 = global read "GVVentilposition.vi" "Ventilposition"() -> (→"Ventilposition":i32)
          n387 = global read "GVZeitenZyklen.vi" "ZyklusNummernGesamt"() -> (→"ZyklusNummernGesamt":i32[])
          n388 = call <vilib>:"RT Get CPU Loads.vi"() -> ("CPU loads"=w968:T25[])  [unwired: 10 in, 1 out]
          n389 = Divide(x=w1060, y=20.0) -> (x/y=w1058:dbl)
          n390 = Divide(x=w1070, y=10.0) -> (x/y=w1068:dbl)
          n391 = Divide(x=w1065, y=10.0) -> (x/y=w1063:dbl)
          n392 = Index Array(array=w968, index=0) -> (element=w966:T25)
          n393 = local read "veränderte Methode benutzen"() -> (w1087:bool)
          n394 = Or(x=w1088, y=w1089) -> (x .or. y?=w1091:bool)
          n395 = Greater Or Equal?(x=w983, y=w988) -> (x >= y?=w986:bool[])
          n396 = Less Or Equal?(x=w983, y=w987) -> (x <= y?=w985:bool[])
          n397 = Greater Or Equal?(x=w974, y=w979) -> (x >= y?=w977:bool[])
          n398 = Less Or Equal?(x=w974, y=w978) -> (x <= y?=w976:bool[])
          n399 = Unbundle(w966) -> ("Total (%)"=→"CPU Total (%)":dbl)  [unwired: 8 out]
          n400 = global read "GVHK1Hz.vi" "Mod1Mod2Mod3/AITrapsMachs1Hz"() -> (w970:dbl[])
          n401 = global write "GVMetavariablen.vi" "MVFixwert"("MVFixwert") -> ()
          n402 = And(x=w986, y=w985) -> (x .and. y?=→"HorstOK?":bool[])
          n403 = And(x=w977, y=w976) -> (x .and. y?=→"MVOK?":bool[])
          n404 = Or(x=w1091, y=w1087) -> (x .or. y?=w1090:bool)
          n405 = global write "GVMetavariablen.vi" "MVFix?"("MVFix?") -> ()
          n406 = global read "GVZeitenZyklen.vi" "Big Ben, Methodenzeit, Zykluszeit0, Zykluszeit1, Zykluszeit2A, Zykluszeit2B"() -> (w1037:dbl[])
          n407 = Array Subset(array=w970, index=0 ("Index"), length=32 ("Länge")) -> (w1021:dbl[])
          "AIs1" <- w1021
          n408 = Array Subset(array=w970, index=32 ("Index"), length=32 ("Länge")) -> (w1009:dbl[])
          "AIs2" <- w1009
          n409 = Array Subset(array=w970, index=96 ("Index"), length=6 ("Länge")) -> (w969:dbl[])
          "schnelle Heizungen" <- w969
          n410 = Array Subset(array=w970, index=64 ("Index"), length=32 ("Länge")) -> (w1000:dbl[])
          "AIs3" <- w1000
          n411 = Greater Or Equal?(x=w969, y=w996) -> (x >= y?=w994:bool[])
          n412 = Less Or Equal?(x=w969, y=w995) -> (x <= y?=w993:bool[])
          n413 = Greater Or Equal?(x=w1021, y=w1022) -> (x >= y?=w1019:bool[])
          n414 = Less Or Equal?(x=w1021, y=w1020) -> (x <= y?=w1018:bool[])
          n415 = Greater Or Equal?(x=w1009, y=w1014) -> (x >= y?=w1012:bool[])
          n416 = Less Or Equal?(x=w1009, y=w1013) -> (x <= y?=w1011:bool[])
          n417 = And(x=w994, y=w993) -> (x .and. y?=→"SHOK?":bool[])
          n418 = Greater Or Equal?(x=w1000, y=w1005) -> (x >= y?=w1003:bool[])
          n419 = Less Or Equal?(x=w1000, y=w1004) -> (x <= y?=w1002:bool[])
          n420 = And(x=w1019, y=w1018) -> (x .and. y?=→"AIs1OK?":bool[])
          n421 = And(x=w1012, y=w1011) -> (x .and. y?=→"AIs2OK?":bool[])
          n422 = And(x=w1003, y=w1002) -> (x .and. y?=→"AIs3OK?":bool[])
          n423 = To Long Integer(number=w1037) -> (32bit integer=→"Big Ben, Methodenzeit, Zykluszeit0, Zykluszeit1, Zykluszeit2A, Zykluszeit2B":i32[])
          n424 = Equal?(x=w1050, y=w1049) -> (x = y?=w1048:bool)
          n425 = call "AnzeigeGV.vi"("veränderte Methode benutzen"=w1087, "Zykluslängen [s]"=w1054, "Cluster1"=w1086, "Big Ben, Methodenzeit, Zykluszeit0, Zykluszeit1, Zykluszeit2A, Zykluszeit2B"=w1037, "Zyklusnummern 0, 1, 2A, 2B"=w1057, "Cluster2"=w1085, "AnzeigeEinstellungen"=w1084, "dargestellte Größe 1"="dargestellte Größe 1", "Zeitachse1"="Zeitachse1", "dargestellte Größe 2"="dargestellte Größe 2", "Zeitachse2"="Zeitachse2") -> ("Anzeige2"=→"Housekeeping2":cluster{dbl[], dbl[]}, "Cluster1"=w1079:cluster{dbl[], dbl[], dbl[], dbl[]}, "x1Inkr"=w1074:dbl, "Cluster2"=w1078:cluster{dbl[], dbl[], dbl[], dbl[]}, "Anzeige1"=→"Housekeeping1":cluster{dbl[], dbl[]}, "AnzeigeEinstellungen"=w1076:T14, "x2Max"=w1038:dbl, "x2Inkr"=w1073:dbl, "x1Max"=w1039:dbl)  [unwired: 8 in]
          n426 = Divide(x=w1052, y=20.0) -> (x/y=w1053:dbl)
          n427 = property on="Detektor 2" class="XYGraph (strikt)"("XScale.Minimum"=w1055, "XScale.Maximum"=w1052, "XScale.Increment"=w1053, "YScale.Minimum"="DetYMin", "YScale.Maximum"="DetYMax", "YScale.Increment"=w1058) -> ()  [unwired: 2 in, 2 out]
          n428 = property on="Housekeeping1" class="XYGraph (strikt)"("XScale.Minimum"=w1055, "XScale.Maximum"=w1039, "XScale.Increment"=w1074, "YScale.Minimum"="HK1YMin", "YScale.Maximum"="HK1YMax", "YScale.Increment"=w1068) -> ()  [unwired: 2 in, 2 out]
          n429 = property on="Housekeeping2" class="XYGraph (strikt)"("XScale.Minimum"=w1055, "XScale.Maximum"=w1038, "XScale.Increment"=w1073, "YScale.Minimum"="HK2YMin", "YScale.Maximum"="HK2YMax", "YScale.Increment"=w1063) -> ()  [unwired: 2 in, 2 out]
          n430 = Select(t=w1046, s=w1048, f=w1047) -> (s? t:f=w1041:cluster{dbl[], dbl[]})
          n431 = Select(t=w1041, s=w1042, f=cluster{dbl[], dbl[]} {[], []} ("s? t:f")) -> (s? t:f=w1034:cluster{dbl[], dbl[]})
          n432 = Build Array(w1045, w1034) -> (→"Detektor 2":cluster{dbl[], "ECD2Chrom":dbl[]}[])
        }
        n433 = while "ZyklusSteuerung" {
          tunnel: w779 -> [w1124]
          tunnel: w780 -> [w1130]
          shift-right: [w1122] -> _
          shift-left: w754 -> [w1128]
          tunnel: w762 -> [w1129]
          tunnel: w680 -> [w1125]
          tunnel: w679 -> [w1126]
          tunnel: w678 -> [w1127]
          shift-right: [w1121] -> _
          shift-left: errorcluster {"status"=FALSE, "code"=0, "source"=""} ("error out") -> [w1123]
          stop <- w1131 stop-if-true
          n434 = call "Bis zum nächsten Vielfachen warten11"("Count(mSec)"=u32 100) -> ()  [unwired: 1 out]
          n435 = global read "GVMethodenwechsel.vi" "Methodenwechsel?"() -> (w1134:bool)
          n436 = global read "gvbooleschRT.vi" "global stop RT"() -> (w1133:bool)
          n437 = local read "veränderte Methode benutzen"() -> (w1132:bool)
          n438 = Compound Arithmetic op=OR(w1134, w1133, w1132) -> (w1131:bool)
          n439 = call "ZyklussteuerungGV-15-07-17.vi"("Traps/MachKoeff0"=w1125, "DIOsNummern"=w1124, "error in"=w1123, "Traps/MachKoeff1"=w1126, "Traps/MachKoeff2"=w1127, "Schieberegister"=w1128, "Zeitpunkte/Setpoints"=w1129, "FPGA VI Reference In"=w1130) -> ("Schieberegister"=w1122:T26, "error out"=w1121:errorcluster)  [unwired: 6 in]
          "Zyklus" <- w1121
        }
        n440 = global read "GVZeitenZyklen.vi" "Big Ben, Methodenzeit, Zykluszeit0, Zykluszeit1, Zykluszeit2A, Zykluszeit2B"() -> (w741:dbl[])
        n441 = Index Array(array=w741, index=3 ("Index")) -> (element=w739:dbl)
        n442 = while {
          tunnel: w783 -> [w907]
          tunnel: w782 -> [w906]
          tunnel: w705 -> [w921]
          shift-right: [w922] -> w776
          shift-left: w781 -> [w923]
          tunnel: w702 -> [w917]
          tunnel: w701 -> [w911]
          shift-right: [w908] -> _
          shift-left: w739 -> [w912]
          stop <- w924 stop-if-true
          n443 = Less?(x=w912, y=w917) -> (x < y?=w915:bool)
          n444 = Less?(x=w912, y=w911) -> (x < y?=w913:bool)
          n445 = call "Bis zum nächsten Vielfachen warten13"("Count(mSec)"=u32 100 ("Zu wartende ms")) -> ()  [unwired: 1 out]
          n446 = global read "GVMethodenwechsel.vi" "Methodenwechsel?"() -> (w926:bool)
          n447 = global read "gvbooleschRT.vi" "global stop RT"() -> (w927:bool)
          n448 = local read "veränderte Methode benutzen"() -> (w925:bool)
          n449 = Compound Arithmetic op=OR(w927, w926, w925) -> (w924:bool)
          n450 = global read "GVZeitenZyklen.vi" "Big Ben, Methodenzeit, Zykluszeit0, Zykluszeit1, Zykluszeit2A, Zykluszeit2B"() -> (w919:dbl[])
          n451 = Index Array(array=w919, index=3 ("Index")) -> (element=w908:dbl)
          n452 = Greater Or Equal?(x=w908, y=w917) -> (x >= y?=w916:bool)
          n453 = Greater Or Equal?(x=w908, y=w911) -> (x >= y?=w914:bool)
          n454 = And(x=w914, y=w913) -> (x .and. y?=w910:bool)
          n455 = And(x=w916, y=w915) -> (x .and. y?=w905:bool)
          n456 = Or(x=w905, y=w910) -> (x .or. y?=w909:bool)
          n457 = And(x=w921, y=w909) -> (x .and. y?=w920:bool)
          n458 = case shown="True" w920 {
            tunnel: w923 -> [w929 w930]
            tunnel: [w929 w934] -> w922
            tunnel: w907 -> [_ w933]
            tunnel: w906 -> [_ w932]
            tunnel: w905 -> [_ w931]
            frame False {
            }
            frame True {
              n459 = call "MSDateienSchicken12-15.vi"("MSNummer"=w930, "MSa?"=w931, "Dateipfad:fromcriordy"=w932, "Dateipfad:fromcriocmd"=w933) -> ()  [unwired: 1 in]
              n460 = Increment(x=w930) -> (x+1=w934:i32)
            }
          }
        }
      }
      n461 = case shown="True" TRUE ("HKSpeichern") {
        tunnel: w417 -> [_ w650]
        frame False {
        }
        frame True {
          n462 = while {
            tunnel: w650 -> [w654]
            shift-right: [w652] -> _
            shift-left: errorcluster {"status"=FALSE, "code"=0, "source"=""} ("error out") -> [w651]
            stop <- w656 stop-if-true
            n463 = call "Bis zum nächsten Vielfachen warten2"("Count(mSec)"=u32 1000) -> ()  [unwired: 1 out]
            n464 = local read "Methode"() -> (w653:i32)
            n465 = global read "gvbooleschRT.vi" "global stop RT"() -> (w656:bool)
            n466 = call "HKinTDMS-01-16.vi"("Methode"=w653, "error in (no error)"=w651, "Kanäle"=w654) -> ("error out"=w652:errorcluster)
            "TDMSwriteHK" <- w652
          }
        }
      }
      n467 = Concatenate Strings("?SE0,GDATA" ("Schreibpuffer"), "\r") -> (w323:string)
      n468 = Build Array(w382, w381, w380) -> (w379:i32[])
      n469 = Add Array Elements(numeric array=w379) -> (sum=w389:i32)
      n470 = Index Array(array=w379, index #1=0 ("Index"), index #2=1 ("Index")) -> (element #1=w400:i32, element #2=w398:i32)
      n471 = while {
        stop <- w1196 stop-if-true
        w1190 = 10.0
        n472 = call "Warten2"("Count(mSec)"=u32 1000) -> ()  [unwired: 1 out]
        n473 = global read "gvbooleschRT.vi" "global stop RT"() -> (w1196:bool)
        n474 = global read "GVTrapsMachs.vi" "Traps/Machs"() -> (w1186:dbl[])
        n475 = global read "GVAIs.vi" "AIs"() -> (w1187:dbl[])
        n476 = for {
          N: 9 -> [_]
          shift-right: [w1199] -> w1193
          shift-left: w1187 -> [w1200]
          shift-right: [w1197] -> w1191
          shift-left: w1186 -> [w1198]
          n477 = flat-sequence {
            tunnel: w1200 -> [w1207]
            tunnel: [w1206] -> w1199
            tunnel: w1198 -> [w1205]
            tunnel: [w1204] -> w1197
            frame #0 {
              n478 = call "Warten28"("Count(mSec)"=u32 100) -> ()  [unwired: 1 out]
            }
            frame #1 {
              n479 = global read "GVAIs.vi" "AIs"() -> (w1203:dbl[])
              n480 = Add(x=w1207, y=w1203) -> (x+y=w1206:dbl[])
              n481 = global read "GVTrapsMachs.vi" "Traps/Machs"() -> (w1202:dbl[])
              n482 = Add(x=w1202, y=w1205) -> (x+y=w1204:dbl[])
            }
          }
        }
        n483 = Divide(x=w1193, y=w1190) -> (x/y=w1192:dbl[])
        n484 = Divide(x=w1191, y=w1190) -> (x/y=w1189:dbl[])
        n485 = Build Array (concatenate)(w1192, w1189) -> (w1188:dbl[])
        n486 = global write "GVHK1Hz.vi" "Mod1Mod2Mod3/AITrapsMachs1Hz"(w1188) -> ()
      }
      n487 = Split 1D Array(array=w378, index=w400) -> (first subarray=w404:dbl[], second subarray=w408:dbl[])
      n488 = Split 1D Array(array=w376, index=w400) -> (first subarray=w407:string[], second subarray=w409:string[])
      n489 = Split 1D Array(array=w377, index=w400) -> (first subarray=w397:string[], second subarray=w399:string[])
      n490 = Initialize Array(-1.0 ("Element"), w389) -> (w374:dbl[])
      n491 = case shown="True" TRUE ("ECDSpeichern") {
        frame False {
        }
        frame True {
          w597 = dbl[] []
          n492 = global read "GVaktuelleTDMS.vi" "aktuelleTDMS-DateiECD1"() -> (w598:refnum<k34>)
          n493 = while {
            shift-right: [w610] -> _
            shift-left: w597 -> [w614]
            shift-right: [w603] -> _
            shift-left: w597 -> [w607]
            shift-right: [w609] -> _
            shift-left: w598 -> [w612]
            tunnel: w597 -> [w606]
            shift-right: [w600] -> _
            shift-left: errorcluster {"status"=FALSE, "code"=0, "source"=""} ("error IO") -> [w599]
            stop <- w619 stop-if-true
            n494 = call "Bis zum nächsten Vielfachen warten3"("Count(mSec)"=u32 500) -> ()  [unwired: 1 out]
            n495 = global read "GVECDs.vi" "ECD1MW"() -> (w613:dbl[])
            n496 = global read "GVECDs.vi" "ECD2MW"() -> (w604:dbl[])
            n497 = global read "gvbooleschRT.vi" "global stop RT"() -> (w619:bool)
            n498 = Build Array (concatenate)(w614, w613) -> (w611:dbl[])
            n499 = Build Array (concatenate)(w607, w604) -> (w608:dbl[])
            n500 = global read "GVaktuelleTDMS.vi" "aktuelleTDMS-DateiECD1"() -> (w609:refnum<k34>)
            n501 = global read "GVaktuelleTDMS.vi" "aktuelleTDMS-DateiECD2"() -> (w617:refnum<k34>)
            n502 = Equal?(x=w612, y=w609) -> (x = y?=w605:bool)
            n503 = TDMS Write(0:w609, 7:"ECD1", 9:w613, 11:w599) -> (15:w602:errorcluster)  [unwired: 2 in, 3 out]
            n504 = TDMS Write(0:w617, 7:"ECD2", 9:w604, 11:w599) -> (15:w601:errorcluster)  [unwired: 2 in, 3 out]
            n505 = Select(t=w611, s=w605, f=w606) -> (s? t:f=w610:dbl[])
            n506 = Select(t=w608, s=w605, f=w606) -> (s? t:f=w603:dbl[])
            n507 = global write "GVChroms.vi" "ECD1Chrom"(w610) -> ()
            n508 = global write "GVChroms.vi" "ECD2Chrom"(w603) -> ()
            n509 = Merge Errors(w602, w601) -> (w600:errorcluster)
            "TDMSwriteECD" <- w600
          }
        }
      }
      n510 = while {
        shift-right: [w426] -> _
        shift-left: w322 -> [w428]
        shift-right: [w425] -> _
        shift-left: w322 -> [w427]
        stop <- w430 stop-if-true
        n511 = call "Bis zum nächsten Vielfachen warten"("Count(mSec)"=u32 100) -> ()  [unwired: 1 out]
        n512 = case shown="True" "An/Aus" {
          tunnel: w428 -> [w432 w448]
          tunnel: w427 -> [w431 w447]
          tunnel: [w432 w441] -> w426
          tunnel: [w431 w440] -> w425
          frame False {
          }
          frame True {
            w444 = dbl[] [] ("t")
            n513 = global read "GVMWHorst.vi" "MWHorst"() -> (w437:dbl[])
            n514 = global read "GVTrapsMachs.vi" "Traps/Machs"() -> (w438:dbl[])
            n515 = Build Array (concatenate)(w438, w437) -> (w436:dbl[])
            n516 = Index Array(array=w436, index="dargestellte Größe 3") -> (element=w449:dbl)
            n517 = Build Array (concatenate)(w448, w449) -> (w442:dbl[])
            n518 = Select(t=w444, s="TafelWischen!", f=w442) -> (s? t:f=w441:dbl[])
            n519 = global read "GVZeitenZyklen.vi" "Big Ben, Methodenzeit, Zykluszeit0, Zykluszeit1, Zykluszeit2A, Zykluszeit2B"() -> (w435:dbl[])
            n520 = Index Array(array=w435, index=1 ("Index")) -> (element=w433:dbl)
            n521 = Build Array (concatenate)(w447, w433) -> (w443:dbl[])
            n522 = Select(t=w444, s="TafelWischen!", f=w443) -> (s? t:f=w440:dbl[])
            n523 = Bundle(w443, w442) -> (→"schnelleAnzeige":cluster{dbl[], dbl[]})  [unwired: 1 in]
          }
        }
        n524 = global read "gvbooleschRT.vi" "global stop RT"() -> (w430:bool)
      }
      n525 = case shown="True" TRUE {
        tunnel: w368 -> [_ w629]
        tunnel: w366 -> [_ w628]
        tunnel: w365 -> [_ w627]
        tunnel: w360 -> [_ w626]
        tunnel: w359 -> [_ w625]
        frame False {
        }
        frame True {
          w620 = errorcluster {"status"=FALSE, "code"=0, "source"=""} ("error out TDMSopen")
          n526 = while {
            shift-right: [w634] -> w624
            shift-left: w626 -> [w636]
            shift-right: [w645] -> w623
            shift-left: w625 -> [w638]
            shift-right: [w640] -> _
            shift-left: w629 -> [w646]
            tunnel: w627 -> [w642]
            tunnel: w628 -> [w643]
            shift-right: [w633] -> w622
            shift-left: w620 -> [w631]
            shift-right: [w632] -> w621
            shift-left: w620 -> [w630]
            stop <- w648 stop-if-true
            n527 = call "Bis zum nächsten Vielfachen warten5"("Count(mSec)"=u32 500) -> ()  [unwired: 1 out]
            n528 = local read "Methode"() -> (w644:i32)
            n529 = global read "gvbooleschRT.vi" "global stop RT"() -> (w648:bool)
            n530 = global read "GVZeitenZyklen.vi" "ZyklusNummernGesamt"() -> (w635:i32[])
            n531 = Index Array(array=w635, index=1 ("Index")) -> (element=w640:i32)
            n532 = Greater?(x=w640, y=w646) -> (0:w639:bool)
            n533 = Select(t=w638, s=w639, f=w636) -> (s? t:f=w637:refnum<k34>)
            n534 = call "AktuelleTDMS.vi"("AktuelleTDMS"=w636, "error in TDMSopen"=w631, "Dateiordner"=w643, "NächsteTDMS"=w638, "NeuerZyklus?"=w639, "Methodennummer"=w644, "Zyklnumges"=w640, "error in TDMSclose"=w630, "Dateiname"=w642) -> ("AktuelleTDMS"=w634:refnum<k34>, "error out TDMSopen"=w633:errorcluster, "error out TDMSclose"=w632:errorcluster, "NächsteTDMS"=w645:refnum<k34>)  [unwired: 3 in]
            "TDMSopenHK" <- w633
            "TDMScloseHK" <- w632
            n535 = global write "GVaktuelleTDMS.vi" "aktuelleTDMS-DateiHK"(w637) -> ()
          }
          n536 = TDMS Close(8:w622, 11:w624) -> ()  [unwired: 2 out]
          n537 = TDMS Close(8:w621, 11:w623) -> ()  [unwired: 2 out]
        }
      }
      n538 = case shown="True" TRUE {
        tunnel: w368 -> [_ w557]
        tunnel: w364 -> [_ w556]
        tunnel: w363 -> [_ w555]
        tunnel: w362 -> [_ w554]
        tunnel: w361 -> [_ w553]
        tunnel: w358 -> [_ w552]
        tunnel: w357 -> [_ w551]
        tunnel: w356 -> [_ w550]
        tunnel: w355 -> [_ w549]
        frame False {
        }
        frame True {
          w542 = errorcluster {"status"=FALSE, "code"=0, "source"=""} ("error out TDMSopen")
          n539 = while {
            shift-right: [w581] -> w548
            shift-left: w552 -> [w583]
            shift-right: [w591] -> w547
            shift-left: w551 -> [w585]
            shift-right: [w589] -> _
            shift-left: w557 -> [w592]
            tunnel: w556 -> [w588]
            tunnel: w554 -> [w587]
            shift-right: [w580] -> w543
            shift-left: w542 -> [w578]
            shift-right: [w579] -> w544
            shift-left: w542 -> [w577]
            stop <- w594 stop-if-true
            n540 = call "Bis zum nächsten Vielfachen warten4"("Count(mSec)"=u32 500) -> ()  [unwired: 1 out]
            n541 = local read "Methode"() -> (w590:i32)
            n542 = global read "gvbooleschRT.vi" "global stop RT"() -> (w594:bool)
            n543 = global read "GVZeitenZyklen.vi" "ZyklusNummernGesamt"() -> (w582:i32[])
            n544 = Index Array(array=w582, index=2 ("Index")) -> (element=w589:i32)
            n545 = Greater?(x=w589, y=w592) -> (0:w586:bool)
            n546 = Select(t=w585, s=w586, f=w583) -> (s? t:f=w584:refnum<k34>)
            n547 = call "AktuelleTDMS.vi"("AktuelleTDMS"=w583, "error in TDMSopen"=w578, "Dateiordner"=w588, "NächsteTDMS"=w585, "NeuerZyklus?"=w586, "Methodennummer"=w590, "Zyklnumges"=w589, "error in TDMSclose"=w577, "Dateiname"=w587) -> ("AktuelleTDMS"=w581:refnum<k34>, "error out TDMSopen"=w580:errorcluster, "error out TDMSclose"=w579:errorcluster, "NächsteTDMS"=w591:refnum<k34>)  [unwired: 3 in]
            "TDMSopenECD1" <- w580
            "TDMScloseECD1" <- w579
            n548 = global write "GVaktuelleTDMS.vi" "aktuelleTDMS-DateiECD1"(w584) -> ()
          }
          n549 = while {
            shift-right: [w571] -> w546
            shift-left: w550 -> [w563]
            shift-right: [w572] -> w545
            shift-left: w549 -> [w565]
            shift-right: [w569] -> _
            shift-left: w557 -> [w573]
            tunnel: w555 -> [w568]
            tunnel: w553 -> [w567]
            shift-right: [w561] -> _
            shift-left: w542 -> [w559]
            shift-right: [w560] -> _
            shift-left: w542 -> [w558]
            stop <- w575 stop-if-true
            n550 = call "Bis zum nächsten Vielfachen warten6"("Count(mSec)"=u32 500) -> ()  [unwired: 1 out]
            n551 = local read "Methode"() -> (w570:i32)
            n552 = global read "gvbooleschRT.vi" "global stop RT"() -> (w575:bool)
            n553 = global read "GVZeitenZyklen.vi" "ZyklusNummernGesamt"() -> (w562:i32[])
            n554 = Index Array(array=w562, index=3 ("Index")) -> (element=w569:i32)
            n555 = Greater?(x=w569, y=w573) -> (0:w566:bool)
            n556 = Select(t=w565, s=w566, f=w563) -> (s? t:f=w564:refnum<k34>)
            n557 = call "AktuelleTDMS.vi"("AktuelleTDMS"=w563, "error in TDMSopen"=w559, "Dateiordner"=w568, "NächsteTDMS"=w565, "NeuerZyklus?"=w566, "Methodennummer"=w570, "Zyklnumges"=w569, "error in TDMSclose"=w558, "Dateiname"=w567) -> ("AktuelleTDMS"=w571:refnum<k34>, "error out TDMSopen"=w561:errorcluster, "error out TDMSclose"=w560:errorcluster, "NächsteTDMS"=w572:refnum<k34>)  [unwired: 3 in]
            "TDMSopenECD2" <- w561
            "TDMScloseECD2" <- w560
            n558 = global write "GVaktuelleTDMS.vi" "aktuelleTDMS-DateiECD2"(w564) -> ()
          }
          n559 = TDMS Close(8:w543, 11:w548) -> ()  [unwired: 2 out]
          n560 = TDMS Close(8:w544, 11:w547) -> ()  [unwired: 2 out]
          n561 = TDMS Close(11:w546) -> ()  [unwired: 1 in, 2 out]
          n562 = TDMS Close(11:w545) -> ()  [unwired: 1 in, 2 out]
        }
      }
      n563 = Split 1D Array(array=w409, index=w398) -> (first subarray=w406:string[], second subarray=w405:string[])
      n564 = Split 1D Array(array=w408, index=w398) -> (first subarray=w403:dbl[], second subarray=w402:dbl[])
      n565 = Split 1D Array(array=w399, index=w398) -> (first subarray=w396:string[], second subarray=w395:string[])
      n566 = Bundle(w407, w406, w405, w404, w403, w402) -> (w401:T27)  [unwired: 1 in]
      n567 = Bundle(w397, w396, w395) -> (w394:cluster{string[], string[], string[]})  [unwired: 1 in]
      n568 = Initialize Array(0.0, 8 ("Dimension")) -> (w324:dbl[])
      n569 = Bundle(w393, w393, w393) -> (w392:cluster{i32, i32, i32})  [unwired: 1 in]
      n570 = Initialize Array("x", 8 ("Dimension")) -> (w329:string[])
      n571 = case shown="True" TRUE ("SerielleKomm.") {
        tunnel: bool[] [TRUE, TRUE, TRUE, TRUE, TRUE, TRUE, TRUE, TRUE] -> [_ w466]
        tunnel: w329 -> [_ w465]
        tunnel: w401 -> [_ w464]
        tunnel: w400 -> [_ w463]
        tunnel: w398 -> [_ w462]
        tunnel: w394 -> [_ w461]
        tunnel: w392 -> [_ w460]
        tunnel: w391 -> [_ w459]
        tunnel: w378 -> [_ w458]
        tunnel: w375 -> [_ w457]
        tunnel: w374 -> [_ w456]
        tunnel: w373 -> [_ w453]
        tunnel: w352 -> [_ w455]
        tunnel: w324 -> [_ w454]
        tunnel: w323 -> [_ w452]
        frame False {
        }
        frame True {
          n572 = while {
            tunnel: w453 -> [w480]
            tunnel: w452 -> [w479]
            shift-right: [w478] -> _
            shift-left: errorcluster {"status"=FALSE, "code"=0, "source"=""} ("error out") -> [w477]
            stop <- w481 stop-if-true
            n573 = call "Warten6"("Count(mSec)"=u32 500) -> ()  [unwired: 1 out]
            n574 = global read "gvbooleschRT.vi" "global stop RT"() -> (w481:bool)
            n575 = case shown="True" "NeuerRefstrom" {
              tunnel: w479 -> [w483 _]
              tunnel: [w482 w492] -> w472
              tunnel: [w482 w495] -> w468
              frame False {
                n576 = String To Byte Array(string=w483) -> (unsigned byte array=w482:u8[])
              }
              frame True {
                n577 = local write "NeuerRefstrom"(FALSE ("NeuerRefstrom")) -> ()
                n578 = Number To Decimal String(number="RefStromECD1", width (-)=i16 4) -> (decimal integer string=w487:string)
                n579 = Number To Decimal String(number="RefStromECD2", width (-)=i16 4) -> (decimal integer string=w484:string)
                n580 = Concatenate Strings("?SE0,SETP," ("string"), w487, "\n") -> (w496:string)
                n581 = Concatenate Strings("?SE0,SETP," ("string"), w484, "\n") -> (w493:string)
                n582 = String To Byte Array(string=w496) -> (unsigned byte array=w495:u8[])
                n583 = String To Byte Array(string=w493) -> (unsigned byte array=w492:u8[])
              }
            }
            n584 = Join Numbers(hi=w468, lo=u8 5) -> ((hi.lo)=w474:u16[])
            n585 = Join Numbers(hi=w472, lo=u8 6) -> ((hi.lo)=w470:u16[])
            n586 = xnode "Invoke Method"("FPGA-VI-Referenz (Eingang)"=w480, "Fehler (Eingang)"=w477, "Daten"=w474) -> ("FPGA-VI-Referenz (Ausgang)"=w473:refnum<k20>, "Fehler (Ausgang)"=w469:errorcluster)  [unwired: 1 in, 1 out]
            n587 = xnode "Invoke Method"("FPGA-VI-Referenz (Eingang)"=w473, "Fehler (Eingang)"=w469, "Daten"=w470) -> ("Fehler (Ausgang)"=w478:errorcluster)  [unwired: 1 in, 2 out]
            "FIFOwriteRS485" <- w478
          }
          n588 = while {
            shift-right: [w499] -> _
            shift-left: w466 -> [w519]
            shift-right: [w523] -> _
            shift-left: w456 -> [w529]
            tunnel: w453 -> [w516]
            shift-right: [w500] -> _
            shift-left: w465 -> [w504]
            tunnel: w457 -> [w507]
            tunnel: w458 -> [w502]
            shift-right: [w508] -> _
            shift-left: w459 -> [w525]
            tunnel: w463 -> [w527]
            tunnel: w462 -> [w528]
            tunnel: w464 -> [w530]
            tunnel: w461 -> [w513]
            shift-right: [w509] -> _
            shift-left: w460 -> [w512]
            shift-right: [w515] -> _
            shift-left: w455 -> [w518]
            shift-right: [w520] -> _
            shift-left: w454 -> [w521]
            shift-right: [w501] -> _
            shift-left: errorcluster {"status"=FALSE, "code"=0, "source"=""} ("error out") -> [w517]
            stop <- w524 stop-if-true
            n589 = for {
              tunnel: w519 -> [w534] mode=indexing
              tunnel: w521 -> [w531] mode=indexing
              tunnel: [w538] -> w520 mode=indexing
              tunnel: [w535] -> w511 mode=indexing
              n590 = global read "GVZeitenZyklen.vi" "Big Ben, Methodenzeit, Zykluszeit0, Zykluszeit1, Zykluszeit2A, Zykluszeit2B"() -> (w541:dbl[])
              n591 = Index Array(array=w541, index=0 ("Index")) -> (element=w539:dbl)
              n592 = Subtract(x=w539, y=w531) -> (x-y=w537:dbl)
              n593 = Greater?(x=w537, y=0.1) -> (0:w533:bool)
              n594 = Or(x=w534, y=w533) -> (x .or. y?=w532:bool)
              n595 = Select(t=w533, s=w533, f=w534) -> (s? t:f=w535:bool)
              n596 = Select(t=w539, s=w532, f=w531) -> (s? t:f=w538:dbl)
            }
            n597 = global read "GVHorstSP.vi" "HorstSP"() -> (w523:dbl[])
            n598 = Not Equal?(x=w523, y=w529) -> (x != y?=w526:bool)
            n599 = call "NeueSP.vi"("Anzahl2"=w528, "Anzahl1"=w527, "AlteSP"=w529, 7:"NeueSP"=w523, "BefehleCluster"=w525, 10:"NeueSP"=w526, "ClusterFest"=w530) -> ("BefehleCluster"=w510:T28)  [unwired: 4 in]
            n600 = call "Warten3"("Count(mSec)"=u32 50) -> ()  [unwired: 1 out]
            n601 = call "MPVSenden-15-07-17.vi"("Ventilposition"=w518, "error in"=w517, "FPGA VI Reference In"=w516) -> ("Ventilposition"=w515:i32, "error out"=w514:errorcluster, "FPGA VI Reference Out"=w506:refnum<k20>)
            n602 = call "Senden-15-07-17.vi"("error in"=w514, "BefehlsCluster"=w510, "AbfragenCluster"=w513, "Abfragenr.Cluster"=w512, "Senden?"=w511, "FPGA VI Reference In"=w506) -> ("BefehlsCluster"=w508:T28, "error out"=w503:errorcluster, "Senden?"=w505:bool[], "Abfragenr.Cluster"=w509:cluster{i32, i32, i32})  [unwired: 1 in]
            n603 = call "SeriellRead-15-07-17.vi"("SkalierungsfaktorHorst"=w502, "VorwortHorst"=w507, "error in"=w503, "Zwischenspeicher"=w504, "Senden?"=w505, "FPGA VI Reference In"=w506) -> ("Senden?"=w499:bool[], "Zwischenspeicher"=w500:string[], "error out"=w501:errorcluster)  [unwired: 3 in]
            "SerielleKomm." <- w501
            n604 = global read "gvbooleschRT.vi" "global stop RT"() -> (w524:bool)
          }
        }
      }
    }
    frame #2 {
      n605 = xnode "Read/Write Control"("FPGA-VI-Referenz (Eingang)"=w1215, "global stop"=TRUE) -> ("FPGA-VI-Referenz (Ausgang)"=w1214:refnum<k20>)  [unwired: 1 in, 1 out]
      n606 = xnode "Close FPGA VI Reference"("FPGA-VI-Referenz (Eingang)"=w1214) -> ()  [unwired: 1 in, 1 out]
    }
    frame #3 {
    }
    frame #4 {
    }
  }
